vi "Main.vi"() -> ()   [LabVIEW 2017]
uses:
  type defs/action buttons.ctl
  type defs/mode buttons.ctl
  <vilib>/vision/Pattern Matching.llb/IMAQ GM Match Report.ctl
  type defs/states.ctl
  type defs/data.ctl
  <vilib>/vision/Image Controls.llb/IMAQ Image.ctl
  <vilib>/myRIO/Instrument Drivers/Onboard IO/PWM/typedefs/PWM Reference.ctl
  <vilib>/myRIO/Common/Instrument Driver Framework/Utilities/typedefs/myRIO Generic Hardware Reference.ctl
  <vilib>/myRIO/Common/Instrument Driver Framework/Utilities/typedefs/Hardware Version Enum.ctl
  <vilib>/myRIO/Common/Instrument Driver Framework/Utilities/typedefs/myRIO v1.0 Reference.ctl
  <vilib>/myRIO/Common/Instrument Driver Framework/Utilities/typedefs/Generic FPGA Reference.ctl
  <vilib>/myRIO/Common/Instrument Driver Framework/myRIO v1.0/PWM/typedefs/PWM Channels Enum.ctl
  <vilib>/myRIO/Instrument Drivers/Onboard IO/PWM/typedefs/PWM Configuration.ctl
  <vilib>/userdefined/High Color/nirio_resource_hc.ctl
  <vilib>/myRIO/Instrument Drivers/Onboard IO/DIO/typedefs/DIO Reference.ctl
  <vilib>/myRIO/Common/Instrument Driver Framework/myRIO v1.0/DIO/typedefs/DIO Channels List.ctl
  <vilib>/myRIO/Common/Instrument Driver Framework/myRIO v1.0/DIO/typedefs/DIO Channels Enum.ctl
  type defs/task.ctl
  <vilib>/myRIO/Common/Instrument Driver Framework/Utilities/vis/Is FPGA Ref Available.vi
  <vilib>/myRIO/Common/Instrument Driver Framework/myRIO v1.0/PWM/vis/myRIO v1.1 Open PWM.vi
  <vilib>/myRIO/Instrument Drivers/Onboard IO/PWM/vis/Set Duty Cycle and Frequency.vi
  <vilib>/myRIO/Common/Instrument Driver Framework/myRIO v1.0/DIO/vis/myRIO v1.1 Open DIO.vi
  <vilib>/myRIO/Instrument Drivers/Onboard IO/DIO/vis/Write.vi
  <vilib>/myRIO/Instrument Drivers/Onboard IO/DIO/vis/Read.vi
  <vilib>/myRIO/Common/Instrument Driver Framework/Utilities/vis/Validate Channels.vi
  <vilib>/myRIO/Common/Instrument Driver Framework/myRIO v1.0/PWM/vis/myRIO v1.0 Reserve PWM.vi
  <vilib>/myRIO/Common/Instrument Driver Framework/myRIO v1.0/DIO/vis/myRIO v1.0 Reserve DIO.vi
  <vilib>/myRIO/Common/Instrument Driver Framework/myRIO v1.0/UART/vis/myRIO v1.0 Close UART.vi
  <vilib>/myRIO/Common/Instrument Driver Framework/myRIO v1.0/PWM/vis/myRIO v1.0 Build MUX Configuration PWM.vi
  <vilib>/myRIO/Common/Instrument Driver Framework/myRIO v1.0/Resource Manager/vis/myRIO v1.0 Reserve Channel List.vi
  <vilib>/myRIO/Common/Instrument Driver Framework/myRIO v1.0/DIO/vis/myRIO v1.0 Build MUX Configuration DIO.vi
  <vilib>/myRIO/Common/Instrument Driver Framework/myRIO v1.0/Resource Manager/vis/myRIO v1.0 Create Configuration List.vi
  <vilib>/myRIO/Common/Instrument Driver Framework/myRIO v1.0/Resource Manager/vis/myRIO v1.0 Reserve Channel.vi
  <vilib>/myRIO/Common/Instrument Driver Framework/myRIO v1.0/Resource Manager/vis/myRIO v1.0 Unreserve Channel.vi
  <vilib>/myRIO/Common/Instrument Driver Framework/myRIO v1.0/Resource Manager/vis/myRIO v1.0 Build Mutex Name.vi
  <vilib>/Utility/VariantDataType/GetNumericInfo.vi
  <vilib>/Utility/error.llb/Error Cluster From Error Code.vi
  <vilib>/myRIO/Common/Instrument Driver Framework/myRIO v1.0/myRIO v1.1 Open.vi
  <vilib>/myRIO/Common/Instrument Driver Framework/Utilities/vis/IO Manager.vi
  <vilib>/myRIO/Common/Instrument Driver Framework/Utilities/vis/Configuration Manager.vi
  <vilib>/myRIO/Common/Instrument Driver Framework/myRIO v1.0/Resource Manager/vis/myRIO v1.0 Configure IO.vi
  <vilib>/myRIO/Common/Instrument Driver Framework/myRIO v1.0/myRIO v1.0 Close.vi
  <vilib>/myRIO/Common/Instrument Driver Framework/myRIO v1.0/PWM/vis/myRIO v1.0 Write PWM.vi
  <vilib>/myRIO/Common/Instrument Driver Framework/myRIO v1.0/DIO/vis/myRIO v1.0 Write DIO.vi
  <vilib>/myRIO/Common/Instrument Driver Framework/myRIO v1.0/DIO/vis/myRIO v1.0 Read DIO.vi
  <vilib>/myRIO/Common/Instrument Driver Framework/Utilities/vis/FPGA Ref Manager.vi
  <vilib>/myRIO/Common/Instrument Driver Framework/myRIO v1.0/myRIO v1.0 Reset FPGA.vi
  <vilib>/myRIO/Common/Instrument Driver Framework/myRIO v1.0/IRQ/vis/myRIO v1.0 IRQ Info FGV.vi
  <vilib>/myRIO/Common/Instrument Driver Framework/myRIO v1.0/IRQ/vis/myRIO v1.0 Timer IRQ Info FGV.vi
  <vilib>/myRIO/Common/Instrument Driver Framework/myRIO v1.0/IRQ/vis/myRIO v1.0 ISR Agent.vi
  <vilib>/myRIO/Express VI/Onboard IO/PWM/PWM Express VI.xnode
  <vilib>/myRIO/Instrument Drivers/Onboard IO/PWM/vis/myRIO PWM Open.xnode
  <vilib>/myRIO/Express VI/Onboard IO/DO/DO Express VI.xnode
  <vilib>/myRIO/Instrument Drivers/Onboard IO/DIO/vis/myRIO DIO Open.xnode
  <vilib>/myRIO/Express VI/Onboard Devices/LED/LED Express VI.xnode
  <vilib>/myRIO/Express VI/Onboard Devices/Button/Button Express VI.xnode
  <vilib>/vision/NI_Vision_Development_Module.lvlib
  <vilib>/myRIO/Instrument Drivers/Onboard IO/DIO/DIO.lvlib
  <vilib>/myRIO/Instrument Drivers/Onboard IO/PWM/PWM.lvlib
  <vilib>/myRIO/Instrument Drivers/Utilities/Utilities.lvlib
panel:
  in  "Ball index":i32
  in  "sensivity":dbl=35000.0 format="%#_13g"
  in  "ROI Descriptor COLOR Mask":T1={"Global Rectangle"=[0, 0, 0, 0], "Contours"=[{"ID"=enum."External", "Type"=0, "Coordinates"=[0, 0, 0, 0]}]}
  out "Radius (circle)":dbl
  out "y0 (circle)":i32
  out "x0 (circle)":i32
  out "x1 (circle)":i32
  out "y1 (circle)":i32
  in  "divider (circle)":sgl=1.0
  out "CircleRadius":dbl
  in  "Look at ball":bool
  in  "x = y?":bool
  in  "y":sgl=1.0
  out "Scale":sgl
  out "error out":errorcluster
  in  "Tab Control":enum32{"Motors", "Shape/Color", "Pattern"}(tab)
  in  "Left+":bool
  in  "Left-":bool
  in  "Right+":bool
  in  "Right-":bool
  in  "M+":bool
  in  "M-":bool
  in  "G+":bool
  in  "G-":bool
  in  "M_PWM":dbl=0.5
  in  "L_PWM":dbl=0.5
  in  "R_PWM":dbl=0.5
  in  "M+ (onGrab)":bool
  out "Circles Calibrated (Shape Detection 1)":T2(array[cluster]) {"Position"."Y" format="%.2f"; "Position"."X" format="%.2f"}
  out "Number of Matches (Shape Detection 1)":i32
  out "Color":i32
  in  "Circle Descriptor (Shape Detection 1)":cluster{"Min Radius":dbl, "Max Radius":dbl}={"Min Radius"=16.0, "Max Radius"=500.0}
  in  "Align X - t, Y - f":bool
  in  "grab time (ms)":u32
  out "Class (Particle Classification 1)":string
  out "y0":i32
  out "x0":i32
  out "x1":i32
  out "y1":i32
  out "Number of Matches (Geometric Matching 1)":i32
  out "Calibrated Matches (Geometric Matching 1)":T3[](array[typedef]) {"Correlation Score" format="%.2f"; "Target Template Curve Score" format="%.2f"; "Template Target Curve Score" format="%.2f"; "Bounding Box"."y" format="%.2f"; "Bounding Box"."x" format="%.2f"; "Position"."y" format="%.2f"; "Position"."x" format="%.2f"; "Score" format="%.2f"; "Scale" format="%.2f"; "Angle" format="%.2f"; "Occlusion %" format="%.2f"}
  out "curY":sgl
  out "curX":sgl
  out "Y is in range":bool
  out "X is in range":bool
  in  "defY":dbl=170.0
  in  "Range":dbl=40.0
  in  "defX":dbl=150.0
  in  "mode buttons":T4
  out "image display":T5(plugin-control)
  in  "action buttons":T6
  in  "Stop":bool
  # "Machine\nVision\nApp"
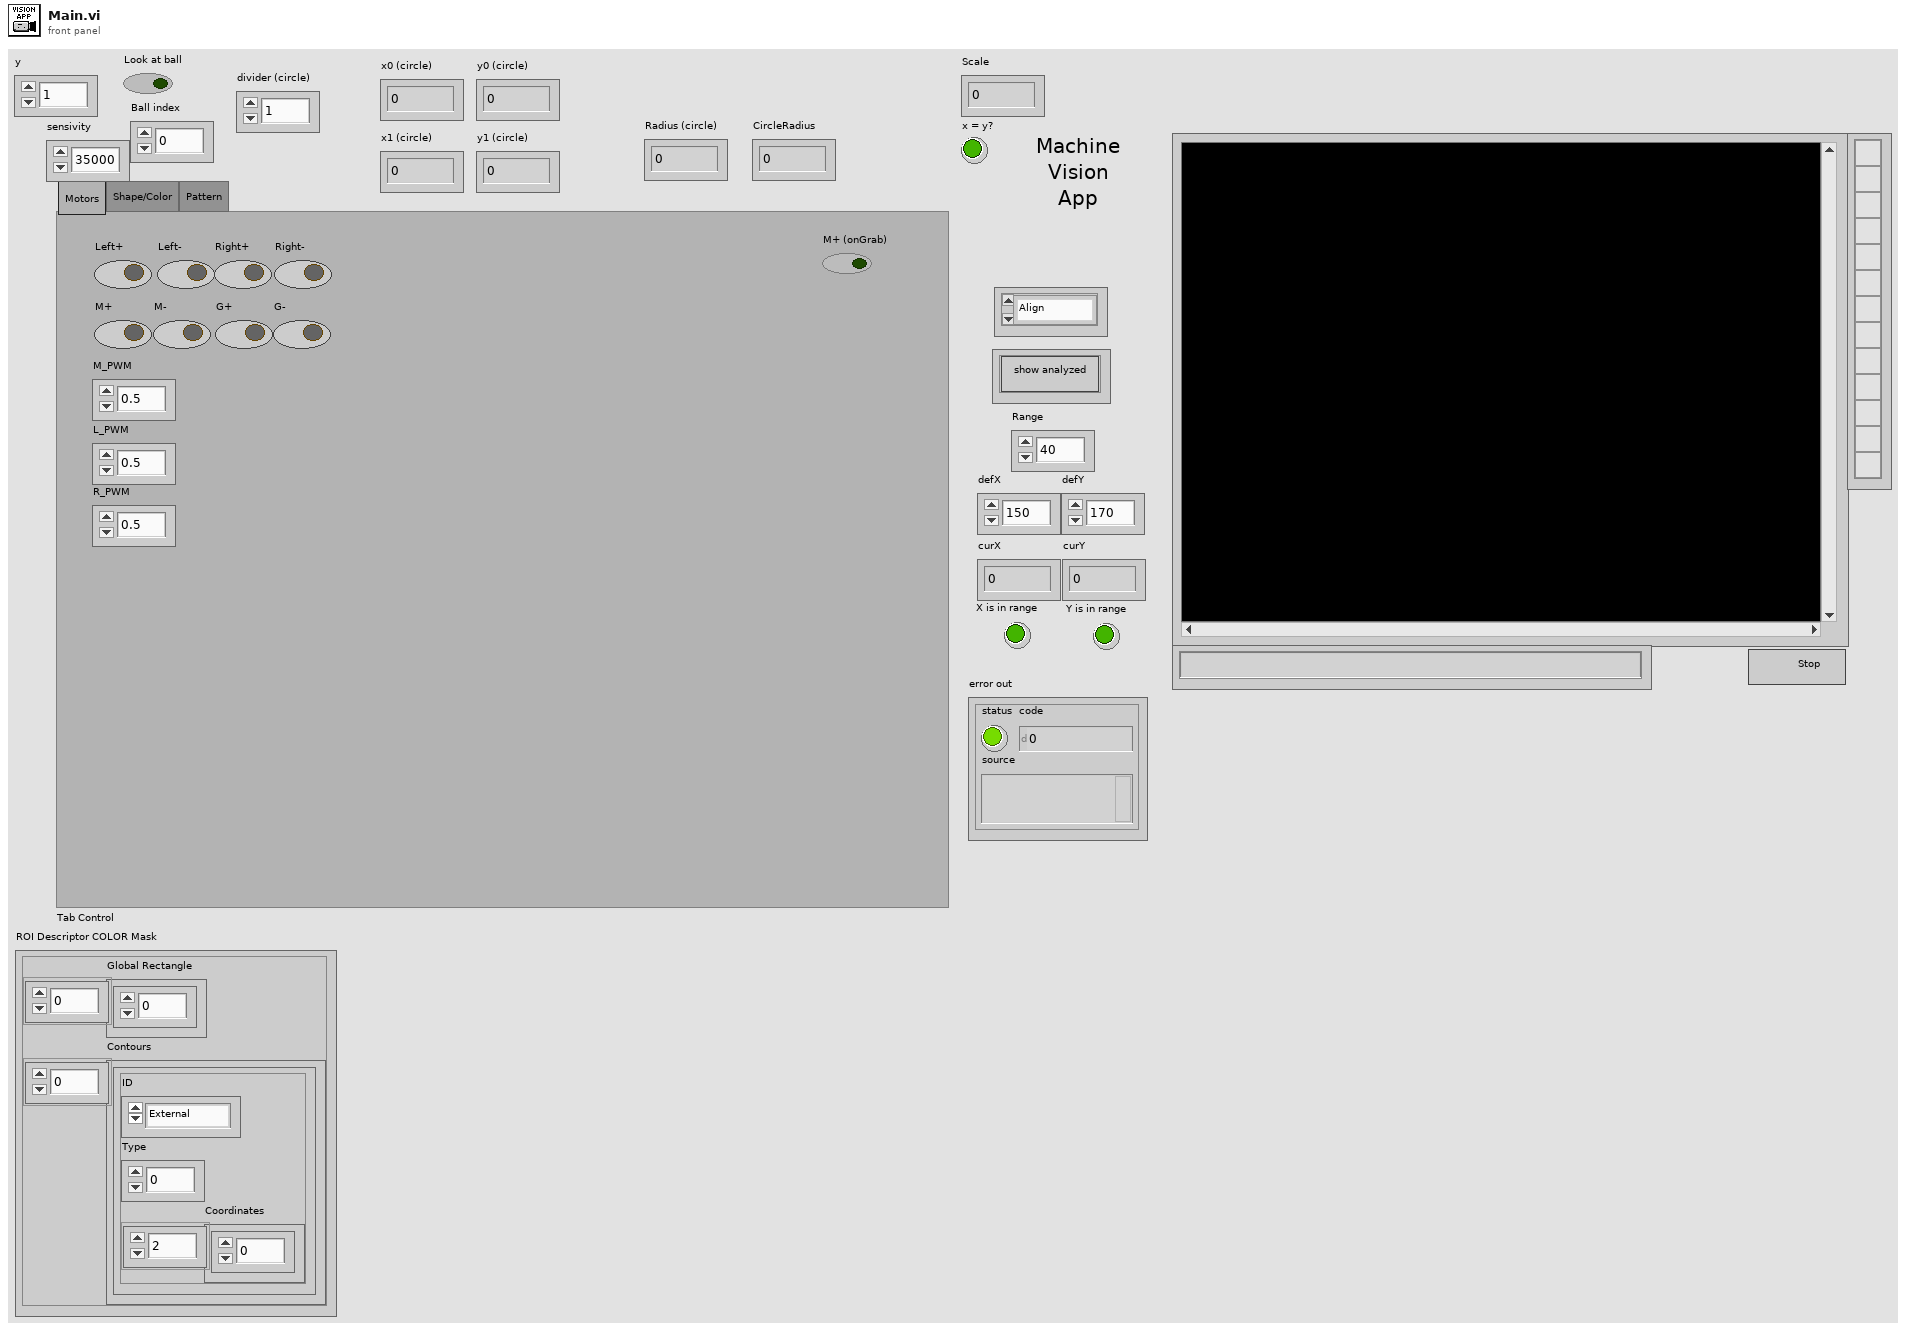
[diagram p1: front panel]
types:
  T1 = cluster{"Global Rectangle":i32[], "Contours":cluster{"ID":enum32{"External", "Internal"}, "Type":u32, "Coordinates":i32[]}[]}
  T2 = cluster{"Position":cluster{"X":sgl, "Y":sgl}, "Radius":dbl, "Score":dbl}[]
  T3 = typedef "IMAQ GM Match Report.ctl" = cluster{"Position":cluster{"x":sgl, "y":sgl}, "Angle":sgl, "Scale":sgl, "Score":sgl, "Bounding Box":cluster{"x":sgl, "y":sgl}[], "Contrast Reversed":bool, "Occlusion %":sgl, "Template Target Curve Score":sgl, "Target Template Curve Score":sgl, "Correlation Score":sgl}
  T4 = typedef "mode buttons.ctl" = cluster{"show analyzed":bool}
  T5 = typedef "IMAQ Image.ctl" = refnum<image>
  T6 = typedef "action buttons.ctl" = cluster{"Shape - t, Color - f":enum16{"Align", "Pattern", "Ball", "Other", "Clear", "Joystick control"}}
  T7 = typedef "states.ctl" = enum16{"(qsm) schedule", "(qsm) initialize", "(qsm) release", "(qsm) clean up", "(qsm) shutdown", "(myRIO) initialize", "(myRIO) clean up", "(myRIO) update ports", "(image) get", "(image) analyze", "(image) show", "(ball) Shape detection", "(ball) Calc ball indx", "(ball) Calculate ROI", "X align", "Wait", "Grab", "(pattern) Find Square", "(pattern) Calculate ROI", "(pattern) Analyze pattern", "(joystick) Joystick control", "Wait for button"}
  T8 = typedef "DIO.lvlib/DIO Reference.ctl" = cluster{"myRIO Reference":T9, "DIO Channels List":T13}
  T9 = typedef "myRIO Generic Hardware Reference.ctl" = cluster{"myRIO Model":T10, "myRIO Hardware Reference":T11}
  T10 = typedef "Hardware Version Enum.ctl" = enum16{"Unknown", "myRIO-1900", "myRIO-1950", "roboRIO", "NI ELVIS RIO CM"}
  T11 = typedef "myRIO v1.0 Reference.ctl" = cluster{"Generic FPGA Reference":T12, "Allow multiple opens":bool}
  T12 = typedef "Generic FPGA Reference.ctl" = refnum<k20>
  T13 = typedef "DIO Channels List.ctl" = T14[]
  T14 = typedef "DIO Channels Enum.ctl" = enum16{"Not Connected", "C/DIO0", "C/DIO1", "C/DIO2", "C/DIO3", "C/DIO4", "C/DIO5", "C/DIO6", "C/DIO7", "A/DIO0", "A/DIO1", "A/DIO2", "A/DIO3", "A/DIO4", "A/DIO5", "A/DIO6", "A/DIO7", "A/DIO8", "A/DIO9", "A/DIO10", "A/DIO11", "A/DIO12", "A/DIO13", "A/DIO14", "A/DIO15", "B/DIO0", "B/DIO1", "B/DIO2", "B/DIO3", "B/DIO4", "B/DIO5", "B/DIO6", "B/DIO7", "B/DIO8", "B/DIO9", "B/DIO10", "B/DIO11", "B/DIO12", "B/DIO13", "B/DIO14", "B/DIO15", "LED0", "LED1", "LED2", "LED3", "Button0", "DIO/DIO0", "DIO/DIO1", "DIO/DIO2", "DIO/DIO3", "DIO/DIO4", "DIO/DIO5", "DIO/DIO6", "DIO/DIO7", "DIO/DIO8", "DIO/DIO9", "SPI/CS0", "SPI/CS1", "SPI/CS2", "SPI/CS3", "LED RADIO (Green)", "LED RADIO (Red)", "LED COMM (Green)", "LED COMM (Red)", "LED MODE (Green)", "LED MODE (Red)"}
  T15 = typedef "nirio_resource_hc.ctl" = tag
  T16 = typedef "PWM.lvlib/PWM Reference.ctl" = cluster{"myRIO Reference":T9, "PWM Channels Enum":T17, "PWM Configuration":T18}
  T17 = typedef "PWM Channels Enum.ctl" = enum16{"Not Connected", "C/PWM0", "C/PWM1", "A/PWM0", "A/PWM1", "A/PWM2", "B/PWM0", "B/PWM1", "B/PWM2", "PWM/PWM0", "PWM/PWM1", "PWM/PWM2", "PWM/PWM3", "PWM/PWM4", "PWM/PWM5", "PWM/PWM6", "PWM/PWM7", "PWM/PWM8", "PWM/PWM9"}
  T18 = typedef "PWM.lvlib/PWM Configuration.ctl" = cluster{"Frequency":dbl, "Duty Cycle":dbl}
  T19 = typedef "data.ctl" = cluster{"Shape - t, Color - f":bool, "qsm":cluster{"Webcam image ref":T5, "Analyzed image ref":T5, "Stop webcam":bool}, " image ref":T5, "number img":i32, "ROI Descriptor (Image Mask 1)":cluster{"Global Rectangle":i32[], "Contours":cluster{"ID":enum32{"External", "Internal"}, "Type":u32, "Coordinates":i32[]}[]}, "Pattern class":i32, "Color class":i32[], "ROI Descriptor COLOR Mask":cluster{"Global Rectangle":i32[], "Contours":cluster{"ID":enum32{"External", "Internal"}, "Type":u32, "Coordinates":i32[]}[]}}
  T20 = enum16{"Align", "Pattern", "Ball", "Other", "Clear", "Joystick control"}
  T21 = typedef "task.ctl" = T7[]
  T22 = typedef "Image Type" = u32
  T23 = cluster{"Position":cluster{"X":sgl, "Y":sgl}, "Radius":dbl, "Score":dbl}
  T24 = cluster{"ID":enum32{"External", "Internal"}, "Type":u32, "Coordinates":i32[]}[]
  T25 = cluster{"ID":enum32{"External", "Internal"}, "Type":u32, "Coordinates":i32[]}
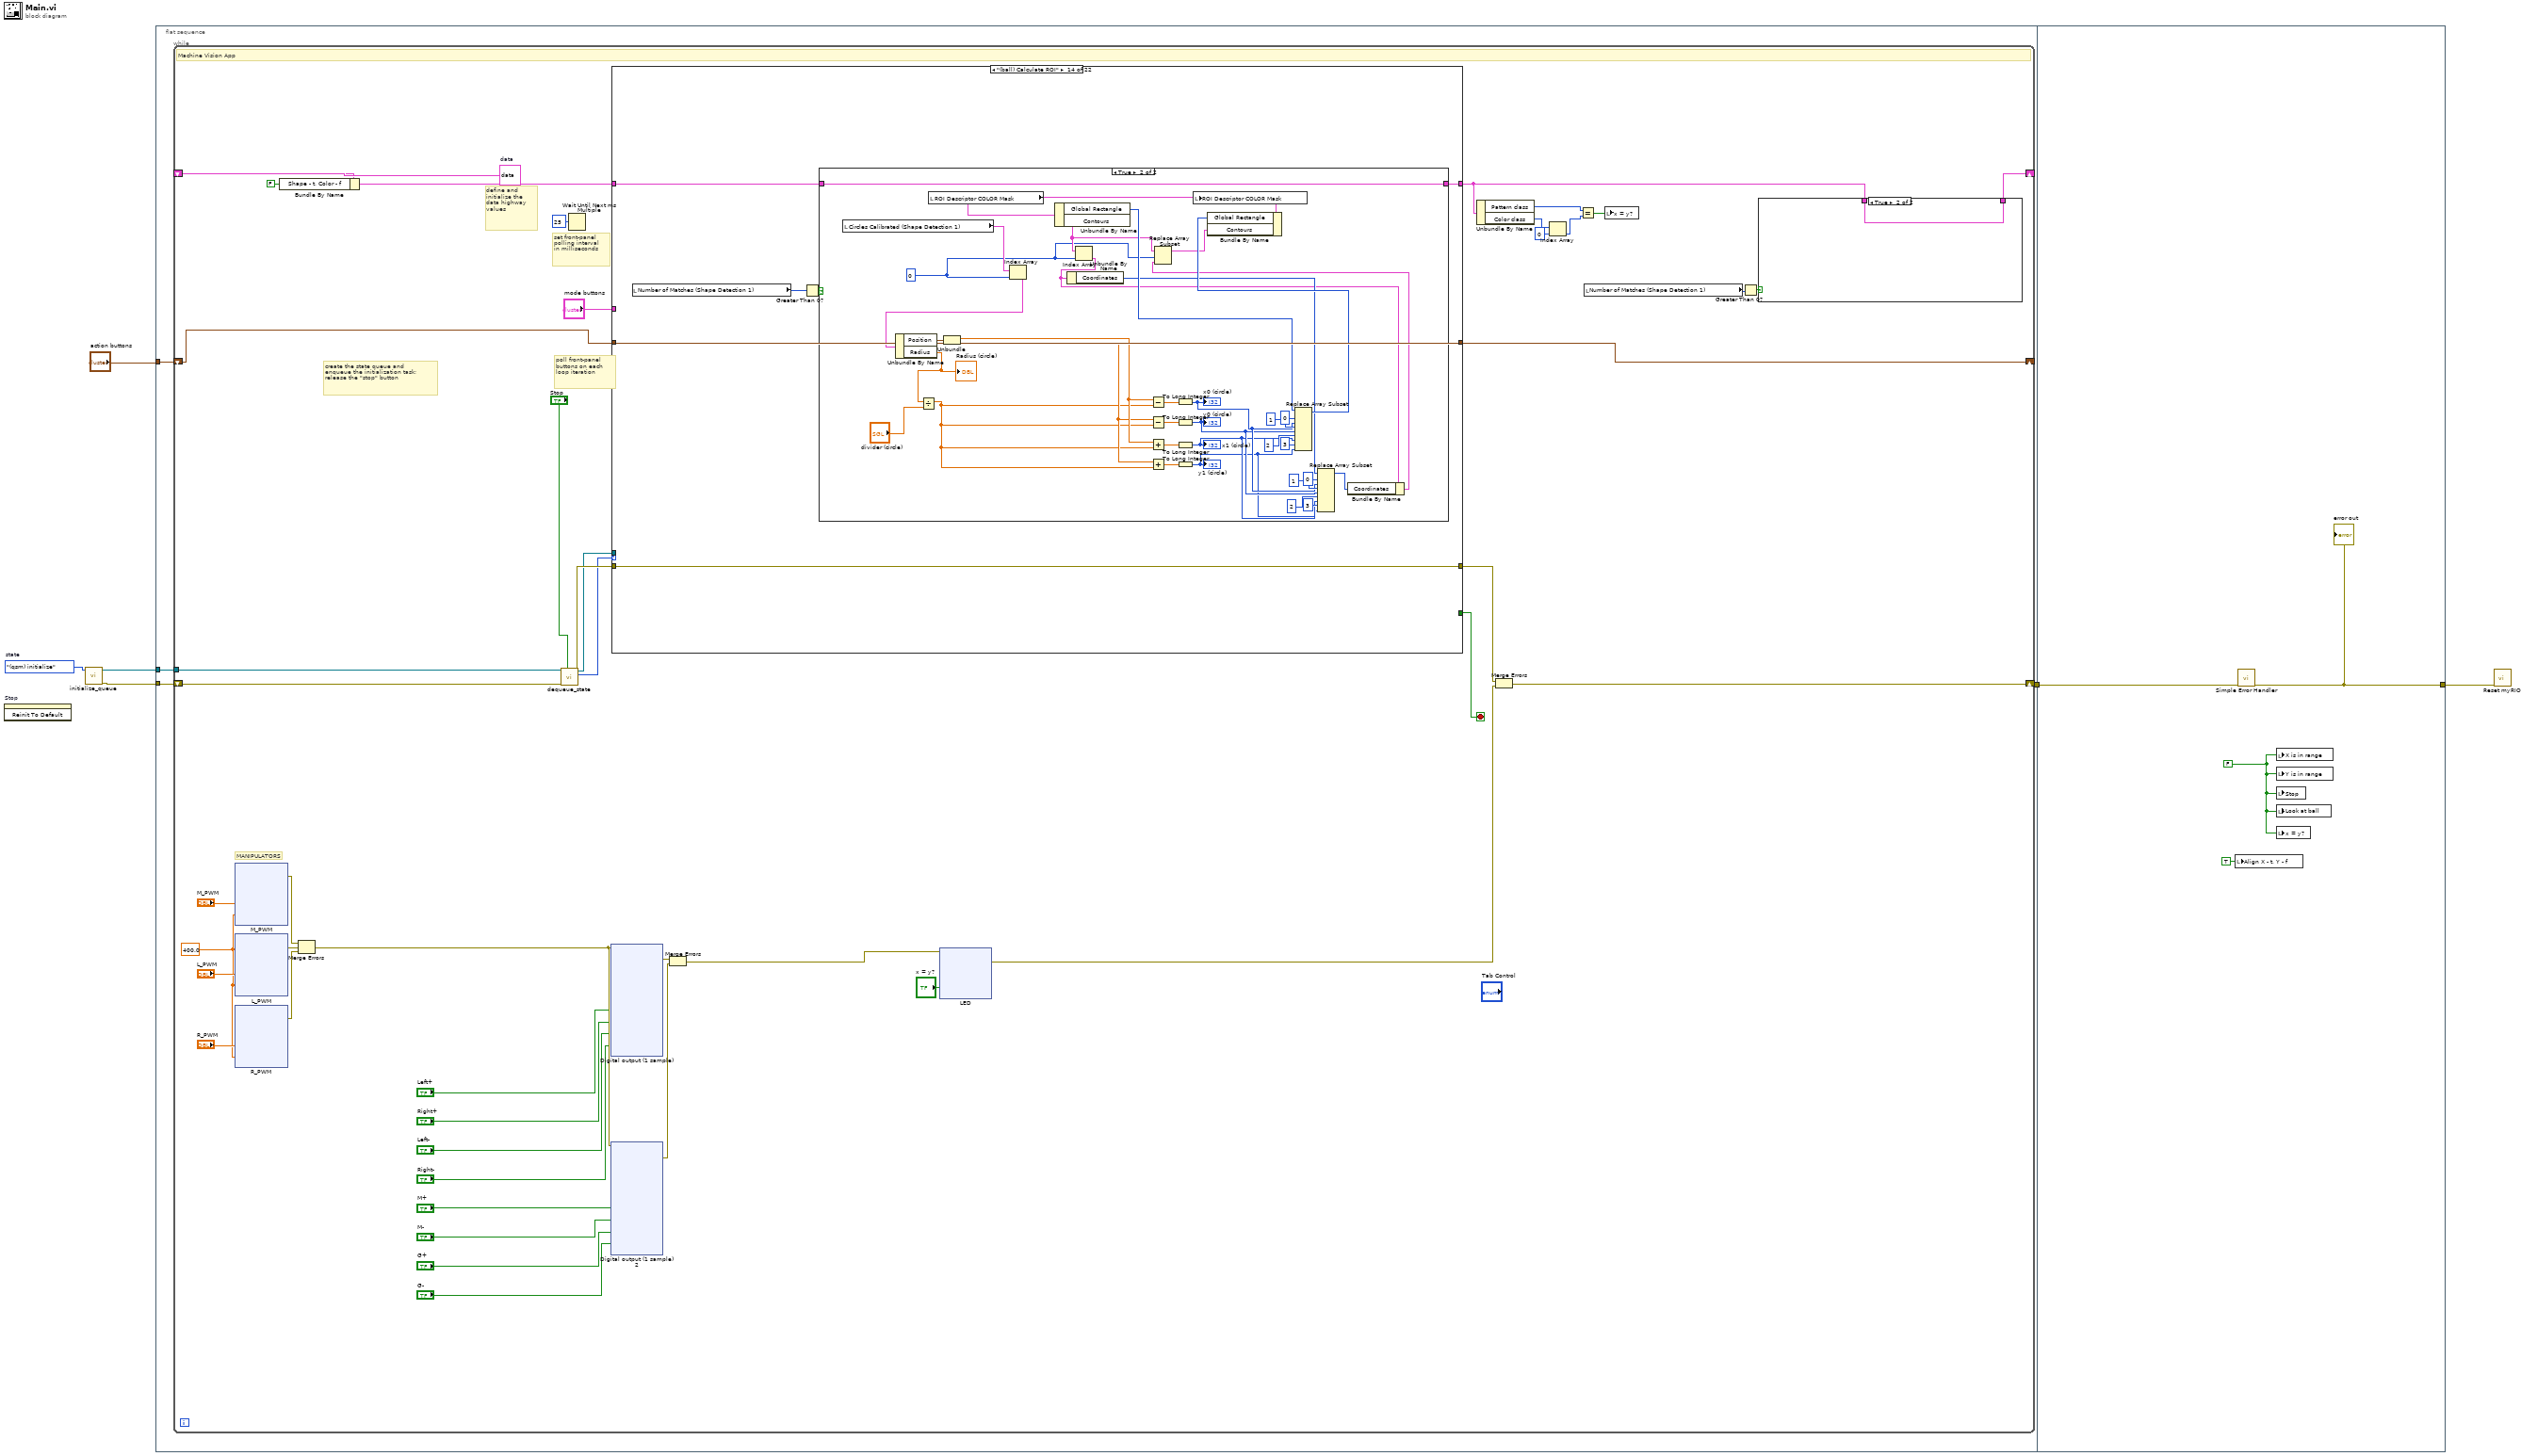
[diagram p0: block diagram]
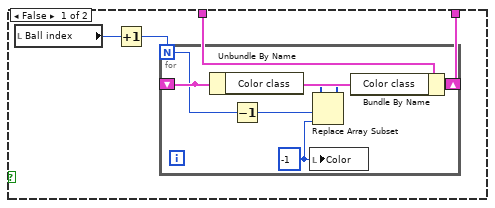
[diagram p2: hidden frame]
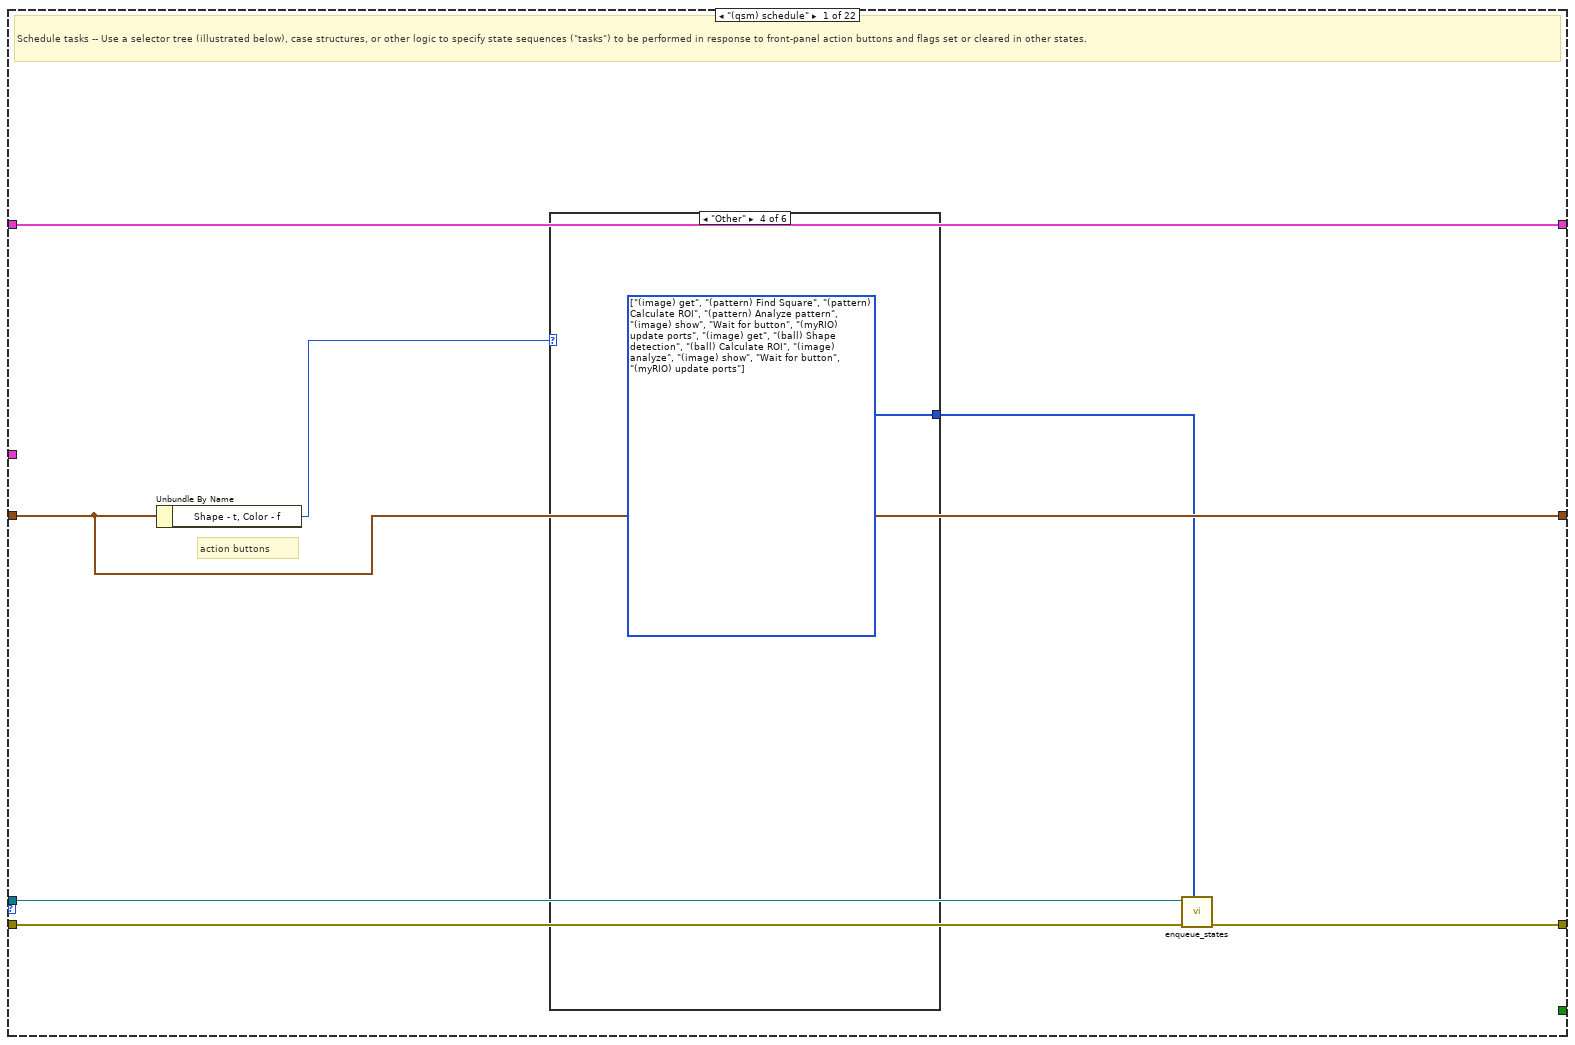
[diagram p3: hidden frame]
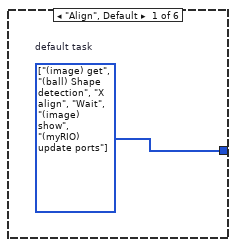
[diagram p4: hidden frame]
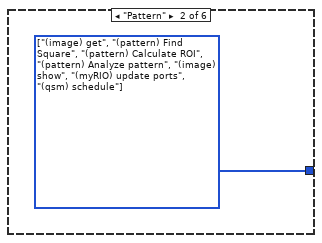
[diagram p5: hidden frame]
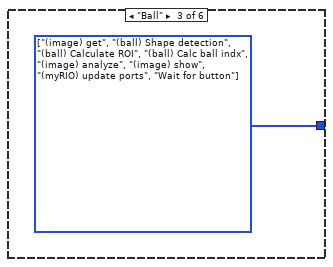
[diagram p6: hidden frame]
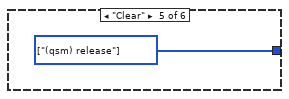
[diagram p7: hidden frame]
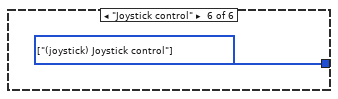
[diagram p8: hidden frame]
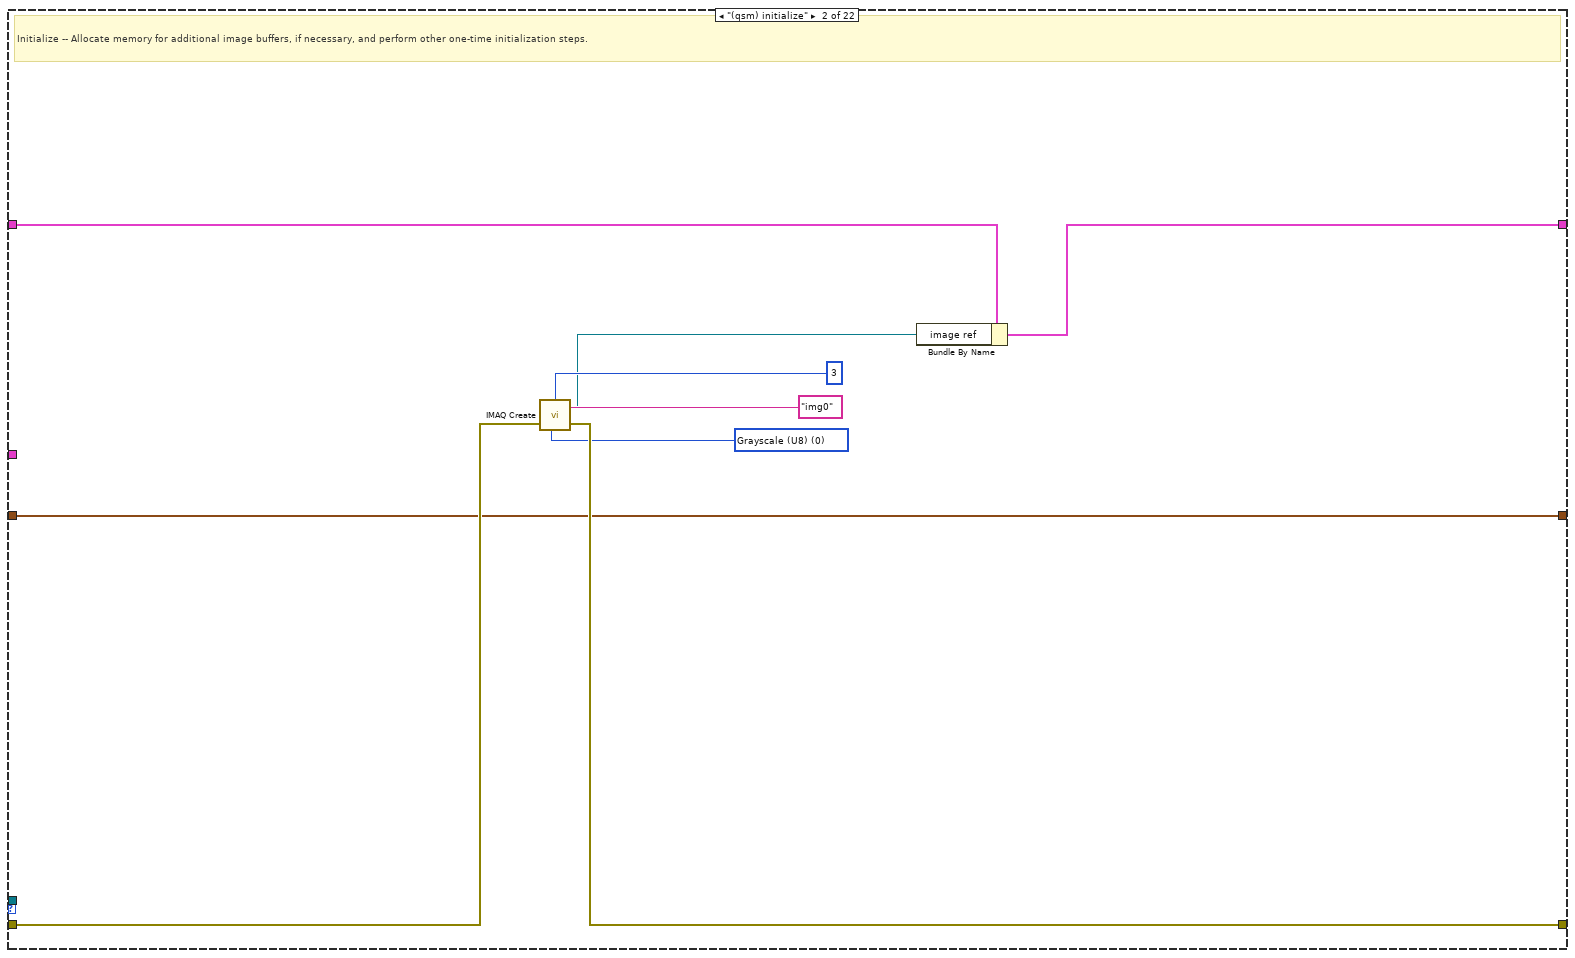
[diagram p9: hidden frame]
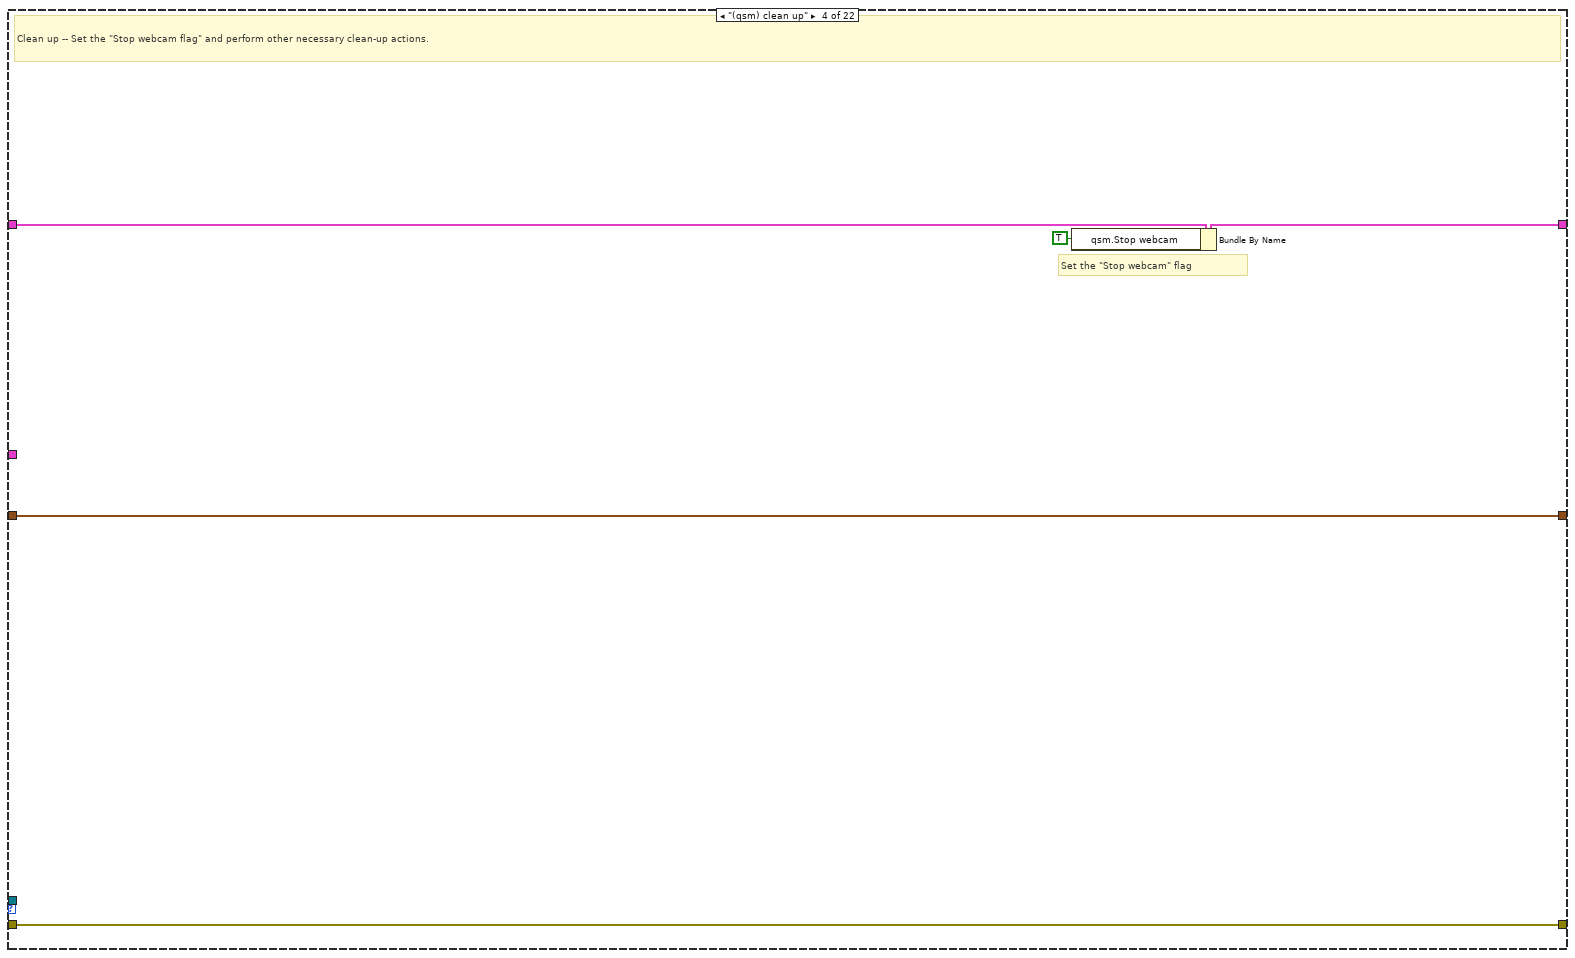
[diagram p11: hidden frame]
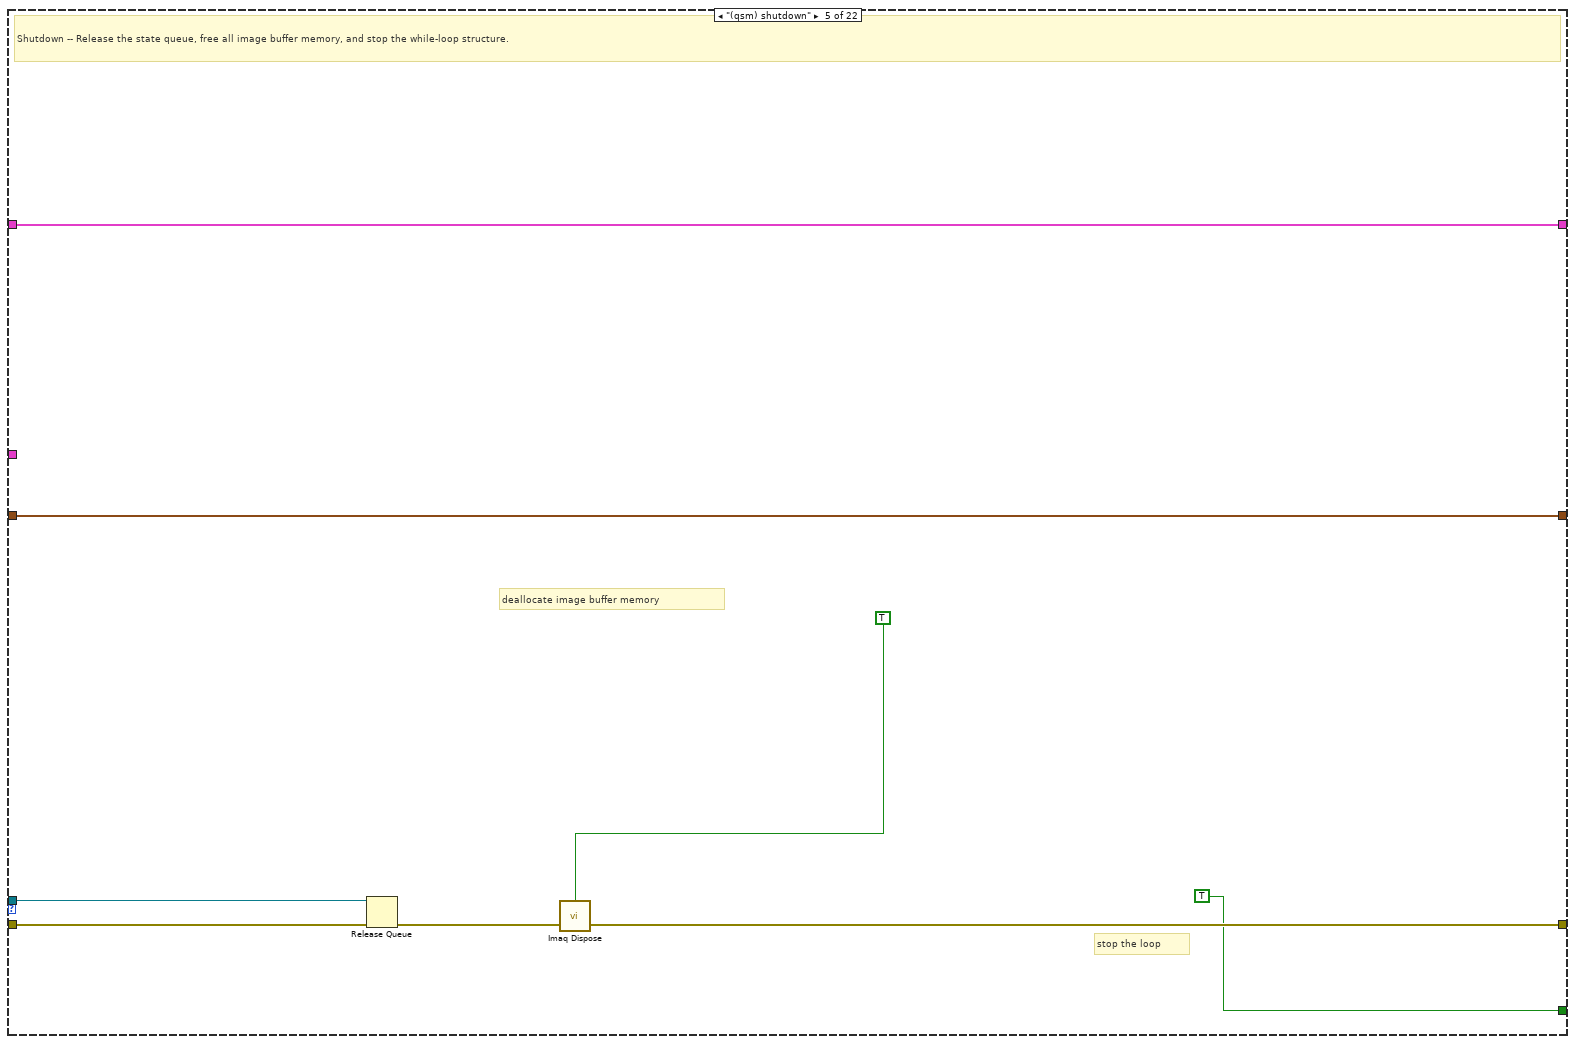
[diagram p12: hidden frame]
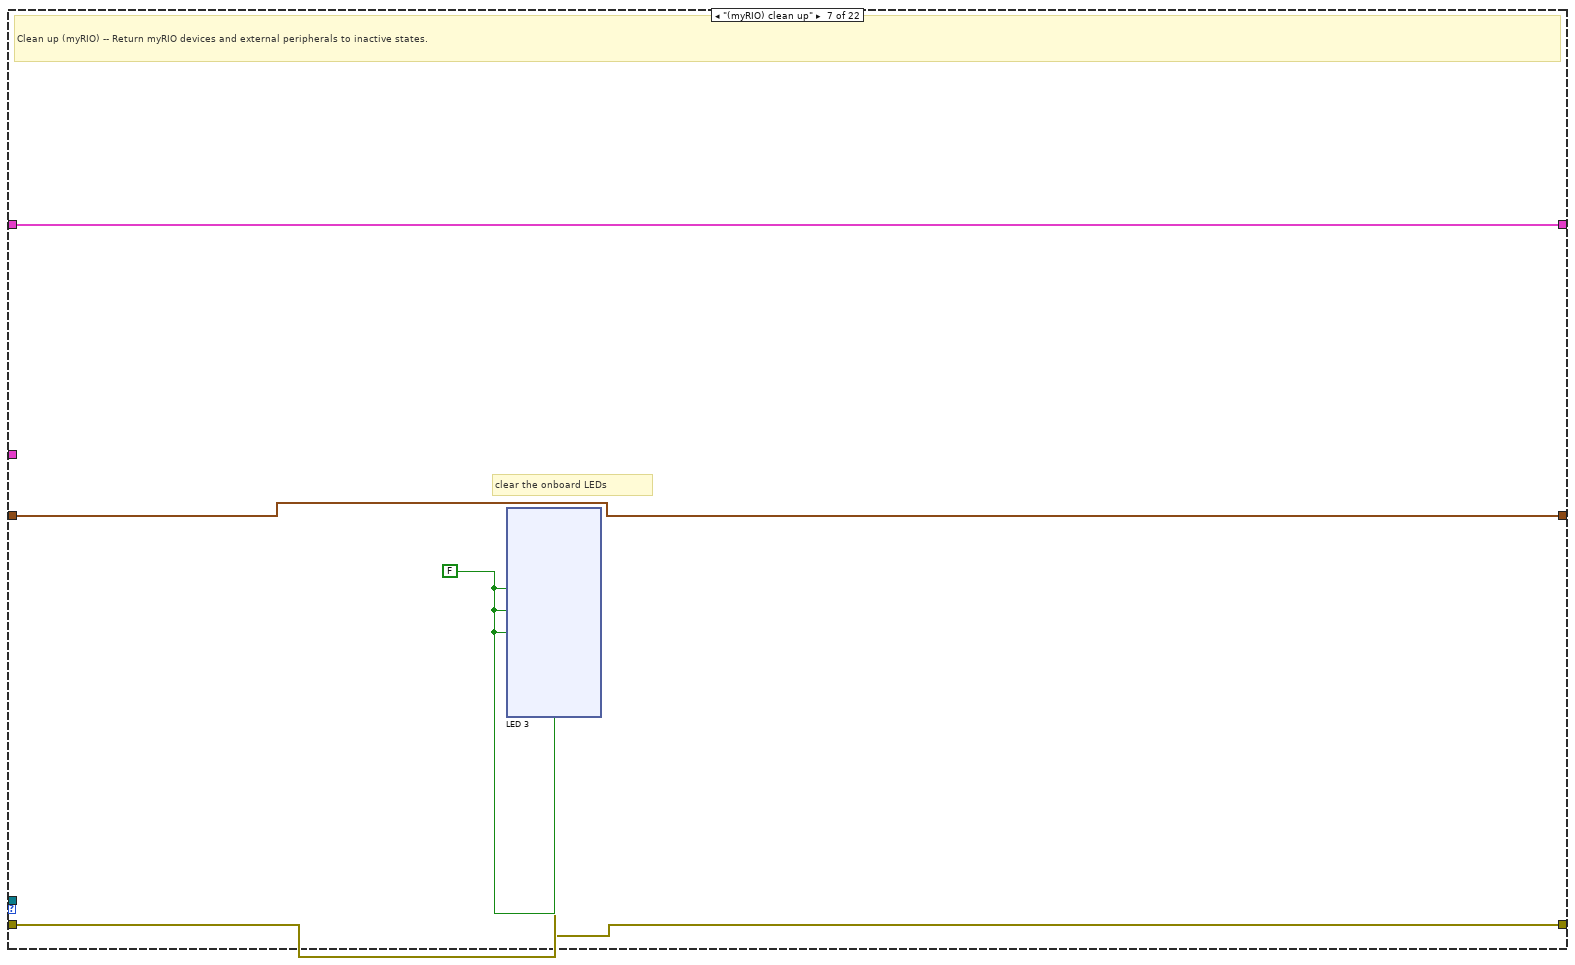
[diagram p14: hidden frame]
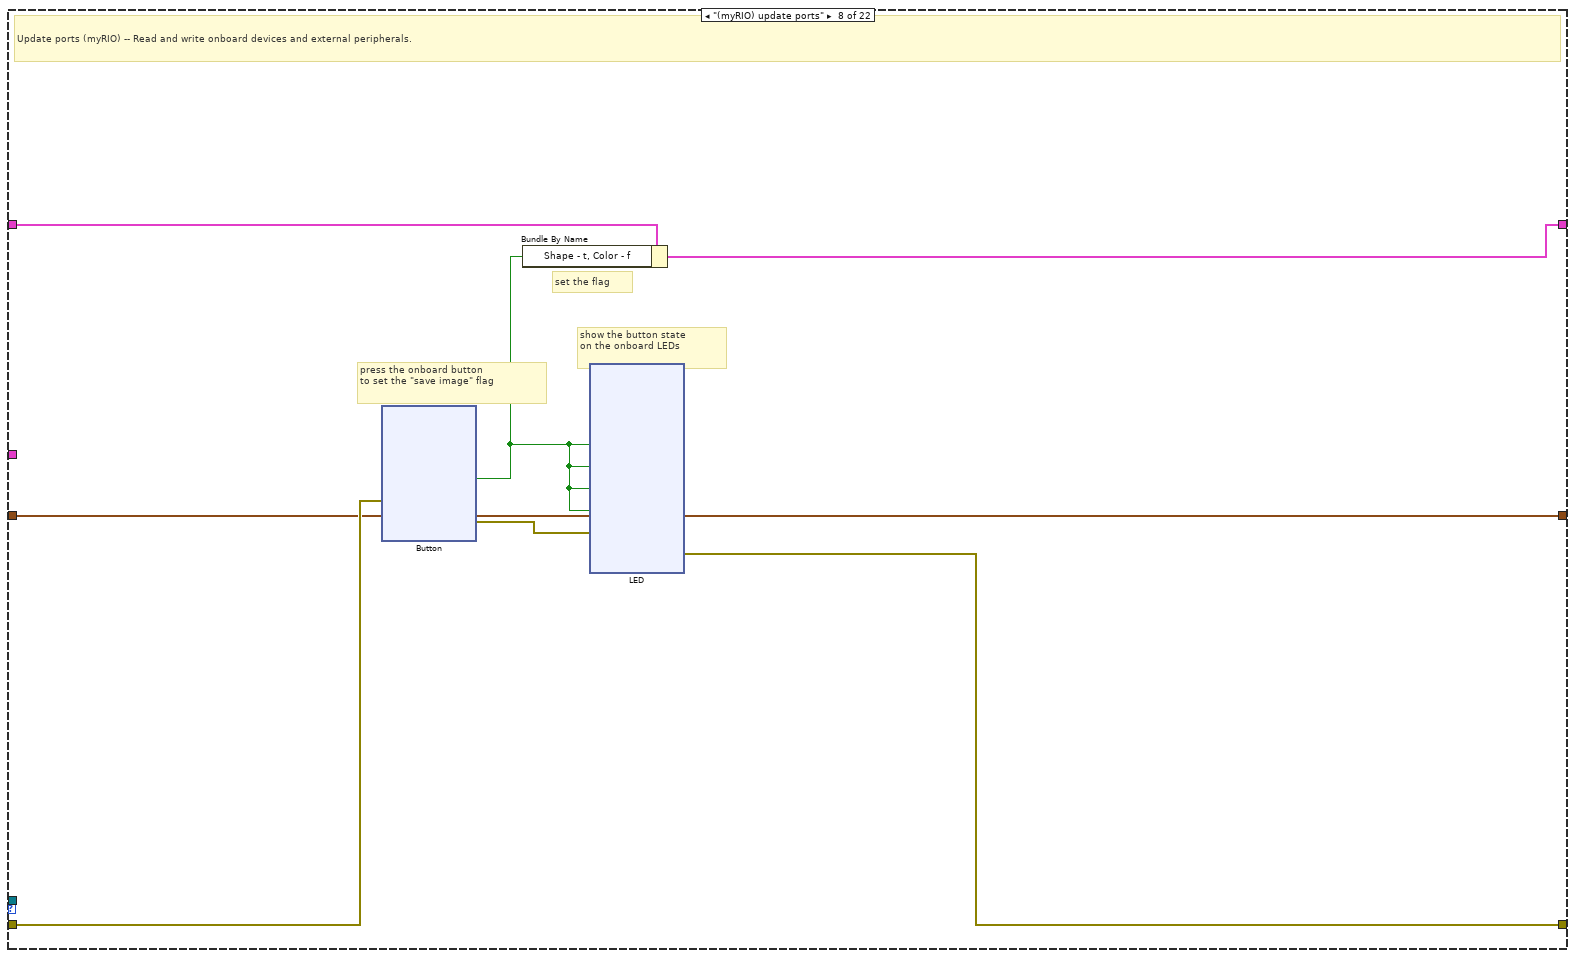
[diagram p15: hidden frame]
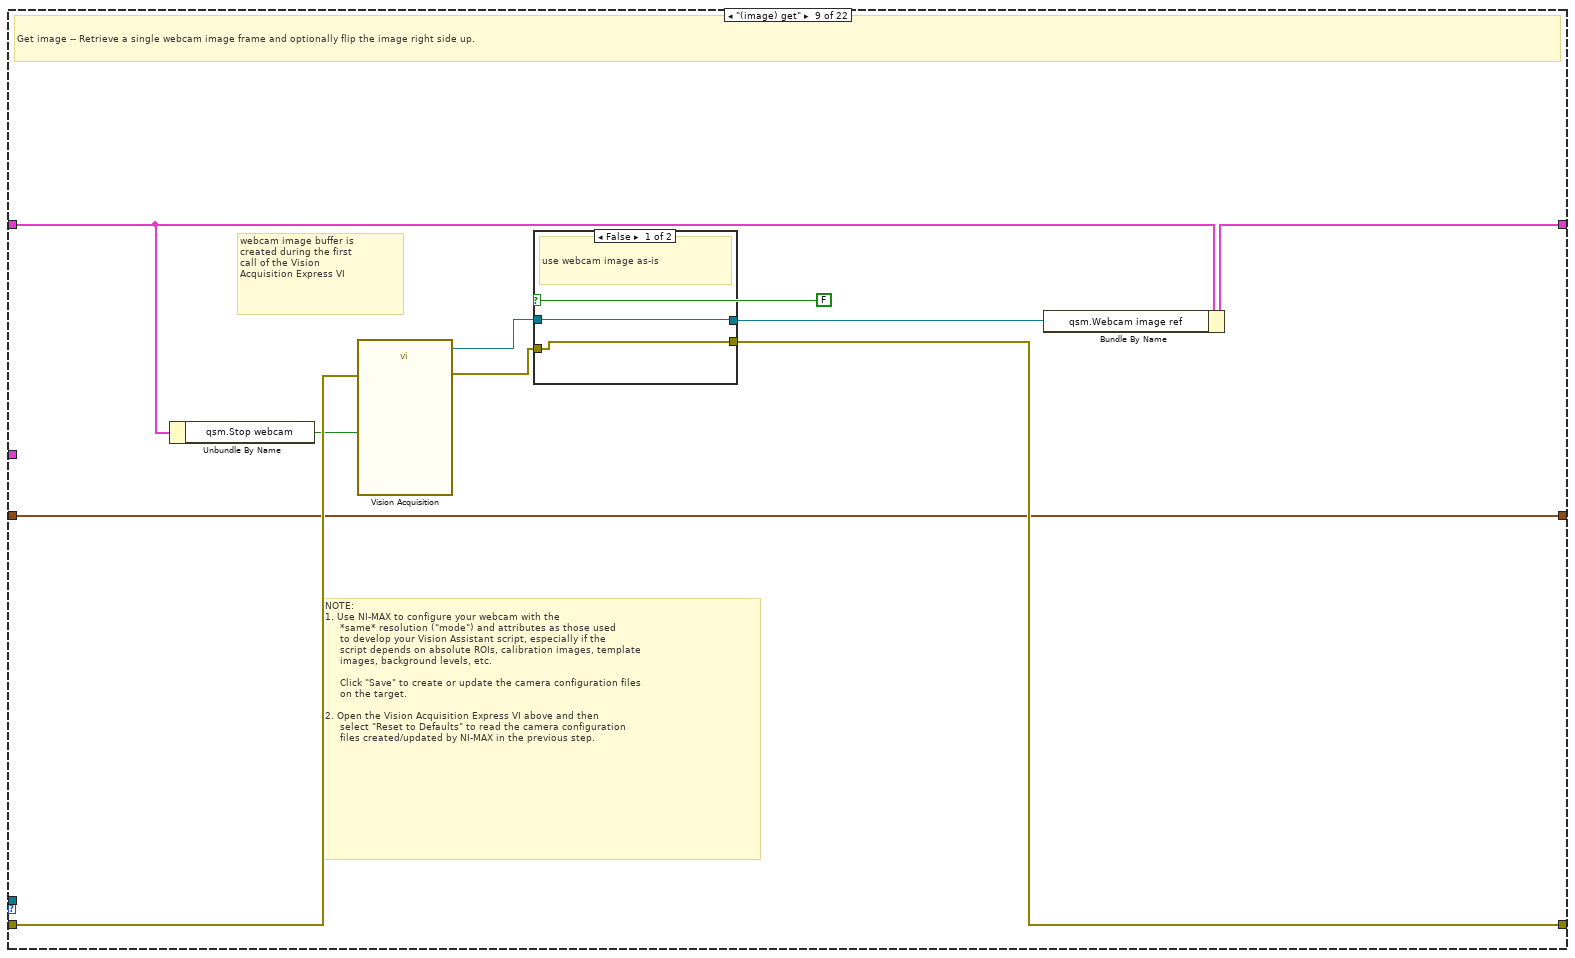
[diagram p16: hidden frame]
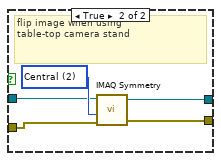
[diagram p17: hidden frame]
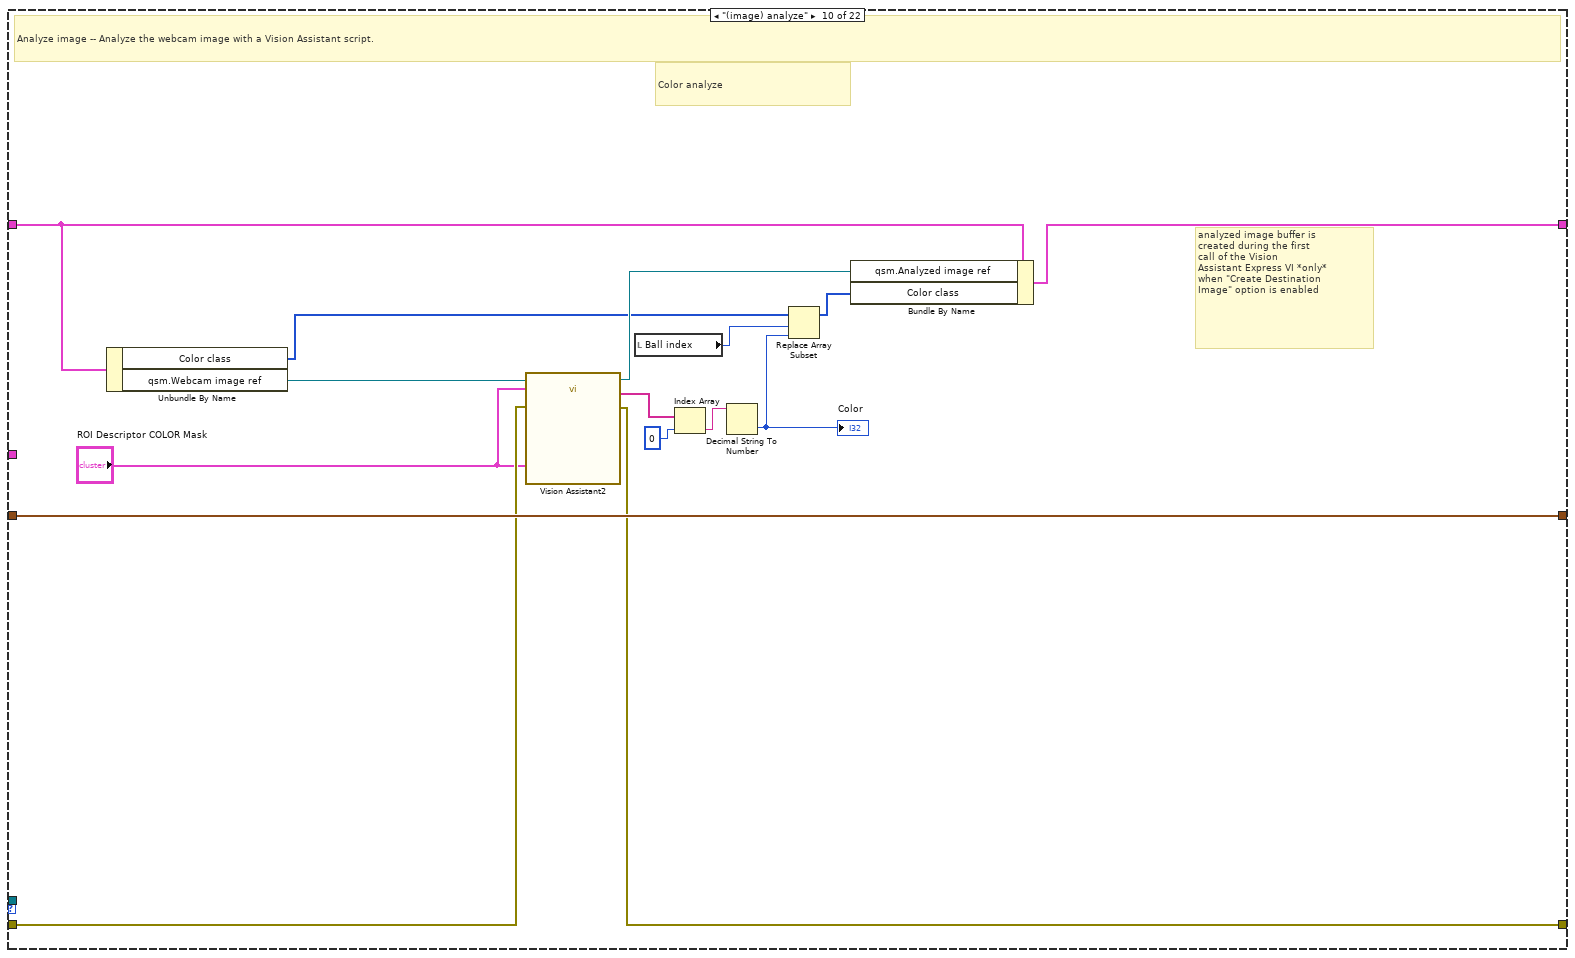
[diagram p18: hidden frame]
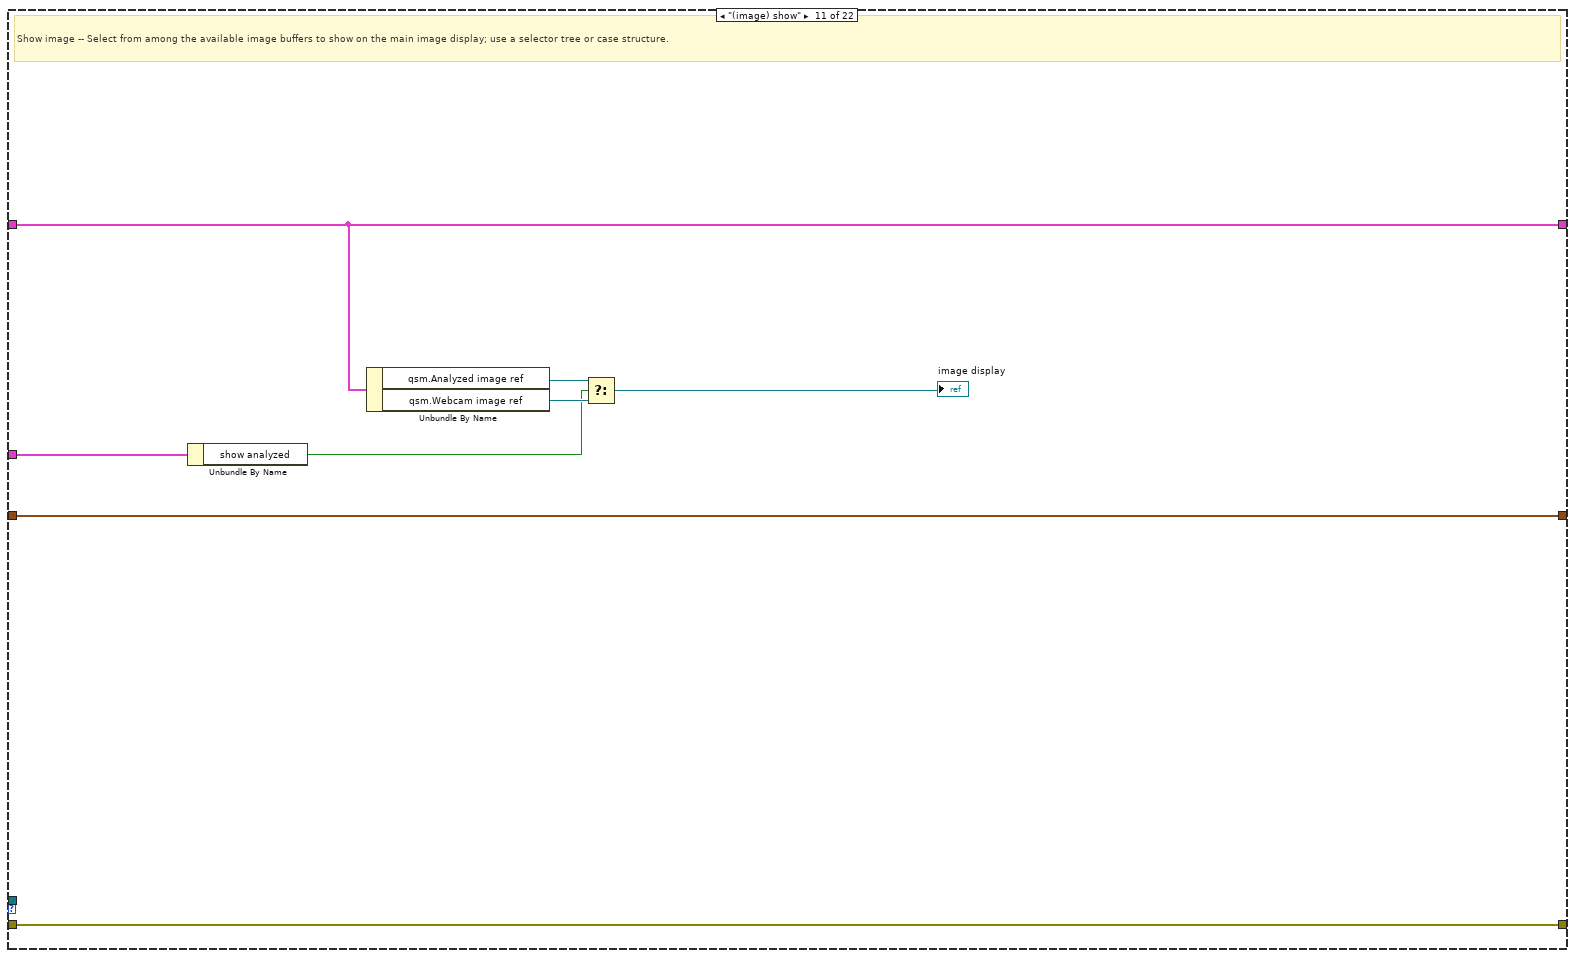
[diagram p19: hidden frame]
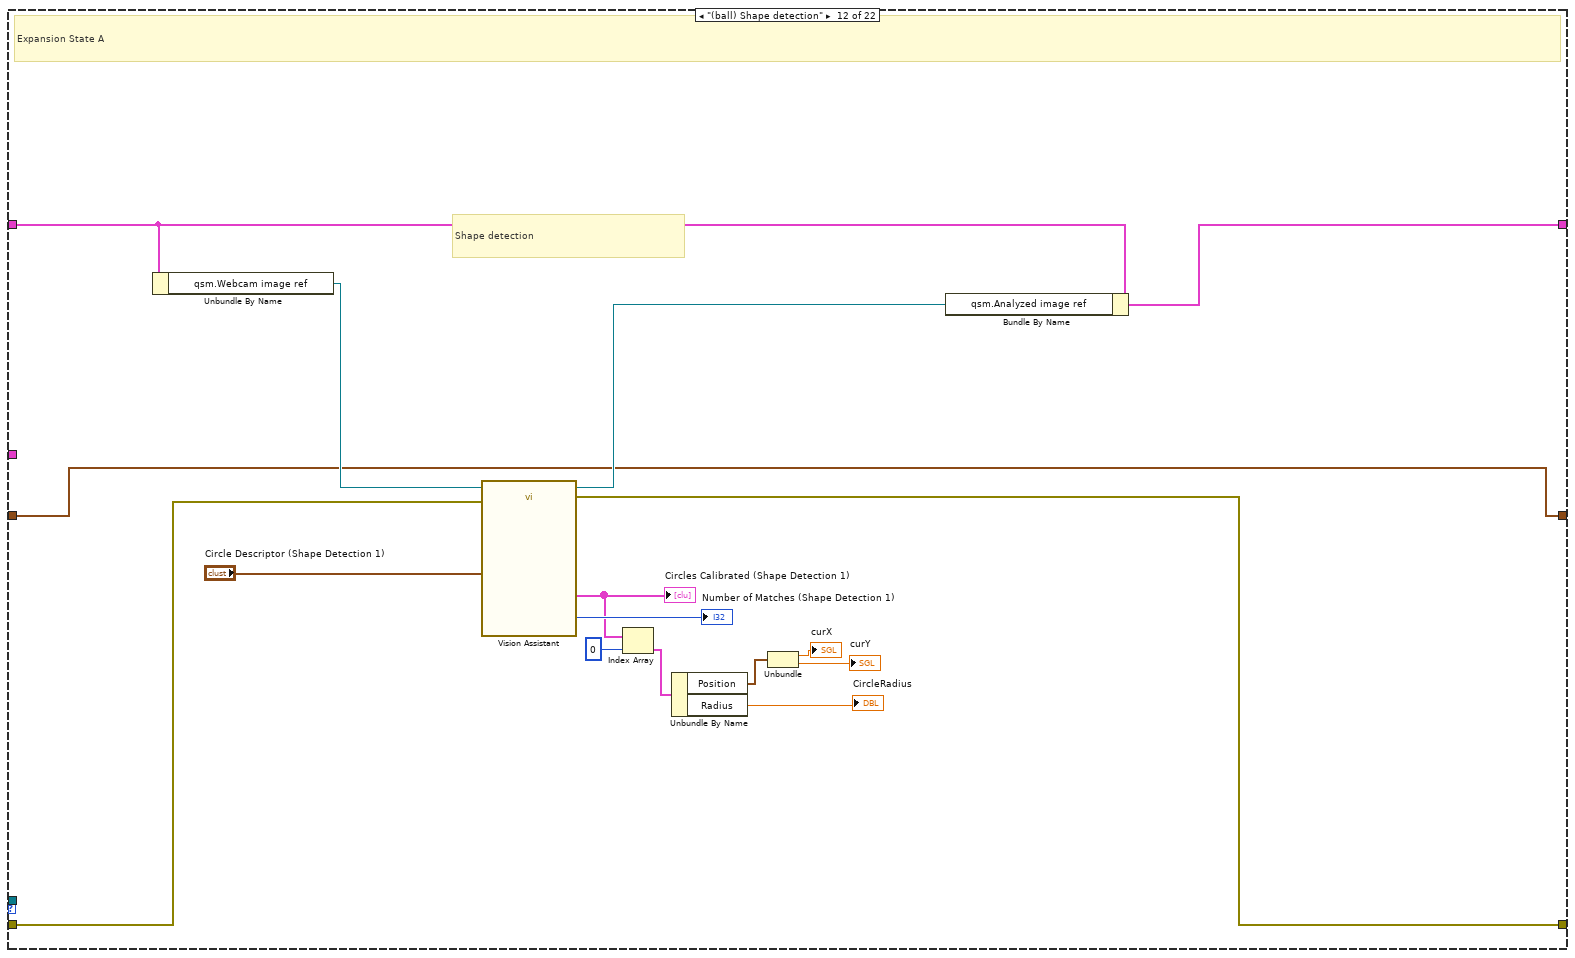
[diagram p20: hidden frame]
diagram:
  w1 = states."(qsm) initialize"  # state
  n1 = invoke on="Stop" class="Bool (strict)" method="Reinit To Default"() -> ()  [unwired: 3 in, 3 out]
  n2 = call "initialize_queue.vi"("state"=w1) -> ("error out"=w2:errorcluster, "queue out"=w3:refnum<queue>)  [unwired: 9 in]
  n3 = flat-sequence {
    tunnel: [w10] -> w5
    tunnel: "action buttons" -> [w9]
    tunnel: w2 -> [w7]
    tunnel: w3 -> [w8]
    tunnel: [w848] -> w6
    tunnel: w5 -> [w849]
    frame #0 {
      w11 = T19 {"Shape - t, Color - f"=FALSE, "qsm"={"Webcam image ref"=refnum, "Analyzed image ref"=refnum, "Stop webcam"=FALSE}, " image ref"=refnum, "number img"=0, "ROI Descriptor (Image Mask 1)"={"Global Rectangle"=[109, 72, 345, 284], "Contours"=[{"ID"=enum."External", "Type"=3, "Coordinates"=[109, 72, 345, 284]}]}, "Pattern class"=0, "Color class"=[], "ROI Descriptor COLOR Mask"={"Global Rectangle"=[51, 157, 345, 350], "Contours"=[{"ID"=enum."External", "Type"=5, "Coordinates"=[137, 230, 93, 226, 75, 199, 49, 200, 56, 145, 98, 111, 200, 119, 250, 126, 235, 166, 240, 212, 188, 243, 303, 244, 336, 247, 336, 271, 335, 292, 335, 318, 314, 323, 293, 334, 279, 345, 272, 349, 187, 349, 186, 335, 120, 334, 112, 314, 100, 297, 59, 291, 51, 288, 51, 287]}]}}  # data
      n4 = while {
        shift-right: [w51] -> w10
        shift-left: w7 -> [w56]
        shift-right: [w18] -> _
        shift-left: w11 -> [w32]
        shift-right: [w31] -> _
        shift-left: w9 -> [w30]
        tunnel: w8 -> [w29]
        stop <- w27 stop-if-true
        w34 = 400.0 ("Frequency [Hz]")
        # "define and \ninitialize the \ndata highway\nvalues"
        # "MANIPULATORS"
        # "create the state queue and\nenqueue the initialization task;\nrelease the \"stop\" button"
        # "set front-panel\npolling interval\nin milliseconds"
        # "poll front-panel\nbuttons on each\nloop iteration"
        # "Machine Vision App"
        n5 = xnode "M_PWM"("Duty Cycle"="M_PWM", "Frequency [Hz]"=w34) -> ("error out"=w50:errorcluster)  [unwired: 1 in]
        n6 = xnode "L_PWM"("Duty Cycle"="L_PWM", "Frequency [Hz]"=w34) -> ("error out"=w49:errorcluster)  [unwired: 1 in]
        n7 = xnode "R_PWM"("Duty Cycle"="R_PWM", "Frequency [Hz]"=w34) -> ("error out"=w48:errorcluster)  [unwired: 1 in]
        n8 = Bundle By Name(cluster=w32, "Shape - t, Color - f"=FALSE) -> (w26:T19)
        n9 = Merge Errors(w50, w49, w48) -> (w45:errorcluster)
        n10 = call "dequeue_state.vi"("stop"="Stop", "error in (no error)"=w56, "queue in"=w29) -> ("error out"=w57:errorcluster, "state"=w52:T7, "queue out"=w33:refnum<queue>)  [unwired: 6 in]
        n11 = Wait Until Next ms Multiple(millisecond multiple=u32 25) -> ()  [unwired: 1 out]
        n12 = xnode "Digital output (1 sample)"("Left+ (A/DIO5 (Pin 21))"="Left+", "Right+ (A/DIO7 (Pin 25))"="Right+", "Left- (A/DIO6 (Pin 23))"="Left-", "Right- (A/DIO13 (Pin 26))"="Right-", "error in (no error)"=w45) -> ("error out"=w47:errorcluster)
        n13 = xnode "Digital output (1 sample) 2"("M+ (B/DIO5 (Pin 21))"="M+", "M- (B/DIO6 (Pin 23))"="M-", "G+ (B/DIO7 (Pin 25))"="G+", "G- (B/DIO13 (Pin 26))"="G-", "error in (no error)"=w45) -> ("error out"=w46:errorcluster)
        n14 = case shown="\"(ball) Calculate ROI\"" w52 {
          tunnel: w57 -> [w289 w307 w309 w312 w323 w325 w329 w374 w454 w472 w485 w505 w507 w517 w582 w618 w637 w720 w730 w786 w822 w842]
          tunnel: w33 -> [w290 _ _ _ w322 _ _ _ _ _ _ _ _ _ w581 w616 _ _ _ _ _ _]
          tunnel: [w291 w306 w309 w312 w318 w325 w328 w372 w457 w473 w485 w500 w507 w517 w582 w617 w636 w721 w730 w785 w822 w842] -> w12
          tunnel: w30 -> [w288 w299 w308 w311 w317 w324 w327 w370 w450 w477 w482 w496 w506 w516 w579 w620 w638 w725 w727 w781 w820 w843]
          tunnel: w26 -> [w292 w301 w310 w314 w321 w326 w331 w376 w455 w481 w486 w502 w508 w519 w583 w622 w639 w719 w728 w784 w821 w844]
          tunnel: [w292 w300 w310 w313 w321 w326 w331 w375 w459 w480 w486 w501 w508 w518 w583 w621 w639 w718 w729 w783 w821 w844] -> w19
          tunnel: "mode buttons" -> [_ _ _ _ _ _ _ _ _ _ w484 _ _ _ _ _ _ _ _ _ _ _]
          tunnel: [w288 w299 w308 w311 w317 w324 w327 w370 w450 w477 w482 w496 w506 w516 w579 w619 w638 w725 w727 w781 w820 w843] -> w31
          tunnel: [_ _ _ _ TRUE _ _ _ _ _ _ _ _ _ _ _ _ _ _ _ _ _] -> w27
          frame "(qsm) schedule" {
            # "action buttons"
            # "Schedule tasks -- Use a selector tree (illustrated below), case structures, or other logic to specify state sequences (\"tasks\") to be performed in response to front-panel action buttons and flags set or cleared in other states."
            n15 = Unbundle By Name(w288) -> ("Shape - t, Color - f"=w287:T20)
            n16 = case shown="\"Other\"" w287 {
              tunnel: [w293 w294 w295 w296 w297 w298] -> w286
              frame "Align", Default {
                w293 = T21 [enum."(image) get", enum."(ball) Shape detection", enum."X align", enum."Wait", enum."(image) show", enum."(myRIO) update ports"] items=["(qsm) schedule", "(qsm) initialize", "(qsm) release", "(qsm) clean up", "(qsm) shutdown", "(myRIO) initialize", "(myRIO) clean up", "(myRIO) update ports", "(image) get", "(image) analyze", "(image) show", "(ball) Shape detection", "(ball) Calc ball indx", "(ball) Calculate ROI", "X align", "Wait", "Grab", "(pattern) Find Square", "(pattern) Calculate ROI", "(pattern) Analyze pattern", "(joystick) Joystick control", "Wait for button"]  # default task
              }
              frame "Pattern" {
                w294 = T21 [enum."(image) get", enum."(pattern) Find Square", enum."(pattern) Calculate ROI", enum."(pattern) Analyze pattern", enum."(image) show", enum."(myRIO) update ports", enum."(qsm) schedule"] items=["(qsm) schedule", "(qsm) initialize", "(qsm) release", "(qsm) clean up", "(qsm) shutdown", "(myRIO) initialize", "(myRIO) clean up", "(myRIO) update ports", "(image) get", "(image) analyze", "(image) show", "(ball) Shape detection", "(ball) Calc ball indx", "(ball) Calculate ROI", "X align", "Wait", "Grab", "(pattern) Find Square", "(pattern) Calculate ROI", "(pattern) Analyze pattern", "(joystick) Joystick control", "Wait for button"] ("task")
              }
              frame "Ball" {
                w295 = T21 [enum."(image) get", enum."(ball) Shape detection", enum."(ball) Calculate ROI", enum."(ball) Calc ball indx", enum."(image) analyze", enum."(image) show", enum."(myRIO) update ports", enum."Wait for button"] items=["(qsm) schedule", "(qsm) initialize", "(qsm) release", "(qsm) clean up", "(qsm) shutdown", "(myRIO) initialize", "(myRIO) clean up", "(myRIO) update ports", "(image) get", "(image) analyze", "(image) show", "(ball) Shape detection", "(ball) Calc ball indx", "(ball) Calculate ROI", "X align", "Wait", "Grab", "(pattern) Find Square", "(pattern) Calculate ROI", "(pattern) Analyze pattern", "(joystick) Joystick control", "Wait for button"] ("task")
              }
              frame "Other" {
                w296 = T21 [enum."(image) get", enum."(pattern) Find Square", enum."(pattern) Calculate ROI", enum."(pattern) Analyze pattern", enum."(image) show", enum."Wait for button", enum."(myRIO) update ports", enum."(image) get", enum."(ball) Shape detection", enum."(ball) Calculate ROI", enum."(image) analyze", enum."(image) show", enum."Wait for button", enum."(myRIO) update ports"] items=["(qsm) schedule", "(qsm) initialize", "(qsm) release", "(qsm) clean up", "(qsm) shutdown", "(myRIO) initialize", "(myRIO) clean up", "(myRIO) update ports", "(image) get", "(image) analyze", "(image) show", "(ball) Shape detection", "(ball) Calc ball indx", "(ball) Calculate ROI", "X align", "Wait", "Grab", "(pattern) Find Square", "(pattern) Calculate ROI", "(pattern) Analyze pattern", "(joystick) Joystick control", "Wait for button"] ("task")
              }
              frame "Clear" {
                w297 = T21 [enum."(qsm) release"] items=["(qsm) schedule", "(qsm) initialize", "(qsm) release", "(qsm) clean up", "(qsm) shutdown", "(myRIO) initialize", "(myRIO) clean up", "(myRIO) update ports", "(image) get", "(image) analyze", "(image) show", "(ball) Shape detection", "(ball) Calc ball indx", "(ball) Calculate ROI", "X align", "Wait", "Grab", "(pattern) Find Square", "(pattern) Calculate ROI", "(pattern) Analyze pattern", "(joystick) Joystick control", "Wait for button"]
              }
              frame "Joystick control" {
                w298 = T21 [enum."(joystick) Joystick control"] items=["(qsm) schedule", "(qsm) initialize", "(qsm) release", "(qsm) clean up", "(qsm) shutdown", "(myRIO) initialize", "(myRIO) clean up", "(myRIO) update ports", "(image) get", "(image) analyze", "(image) show", "(ball) Shape detection", "(ball) Calc ball indx", "(ball) Calculate ROI", "X align", "Wait", "Grab", "(pattern) Find Square", "(pattern) Calculate ROI", "(pattern) Analyze pattern", "(joystick) Joystick control", "Wait for button"]
              }
            }
            n17 = call "enqueue_states.vi"("task"=w286, "error in"=w289, "queue in"=w290) -> ("error out"=w291:errorcluster)  [unwired: 6 in, 1 out]
          }
          frame "(qsm) initialize" {
            w304 = T22 0 items=["Grayscale (U8)", "Grayscale (I16)", "Grayscale (SGL)", "Complex (CSG)", "RGB (U32)", "HSL (U32)", "RGB (U64)", "Grayscale (U16)"] ("Image Type")
            # "Initialize -- Allocate memory for additional image buffers, if necessary, and perform other one-time initialization steps."
            n18 = call "IMAQ Create"("Border Size"=3, "Image Name"="img0", "Image Type"=w304, "error in (no error)"=w307) -> ("New Image"=w302:T5, "error out"=w306:errorcluster)  [unwired: 1 in]
            n19 = Bundle By Name(cluster=w301, "image ref"=w302) -> (w300:T19)
          }
          frame "(qsm) release" {
            # "Release all front-panel action buttons."
          }
          frame "(qsm) clean up" {
            # "Set the \"Stop webcam\" flag"
            # "Clean up -- Set the \"Stop webcam flag\" and perform other necessary clean-up actions."
            n20 = Bundle By Name(cluster=w314, "qsm.Stop webcam"=TRUE) -> (w313:T19)
          }
          frame "(qsm) shutdown" {
            # "deallocate image buffer memory"
            # "stop the loop"
            # "Shutdown -- Release the state queue, free all image buffer memory, and stop the while-loop structure."
            n21 = Release Queue(queue=w322, error in (no error)=w323) -> (error out=w319:errorcluster)  [unwired: 1 in, 2 out]
            n22 = call "Imaq Dispose"("All Images? (No)"=TRUE, "error in (no error)"=w319) -> ("error out"=w318:errorcluster)  [unwired: 4 in]
          }
          frame "(myRIO) initialize" {
            # "Initialize (myRIO) -- Open channels, configure devices, send setup strings to peripherals, etc."
          }
          frame "(myRIO) clean up" {
            w330 = FALSE ("LED3")
            # "clear the onboard LEDs"
            # "Clean up (myRIO) -- Return myRIO devices and external peripherals to inactive states."
            n23 = xnode "LED 3"("LED0"=w330, "LED1"=w330, "LED2"=w330, "LED3"=w330, "error in (no error)"=w329) -> ("error out"=w328:errorcluster)
          }
          frame "(myRIO) update ports" {
            # "show the button state\non the onboard LEDs"
            # "set the flag"
            # "press the onboard button\nto set the \"save image\" flag"
            # "Update ports (myRIO) -- Read and write onboard devices and external peripherals."
            n24 = xnode "Button"("error in (no error)"=w374) -> ("Value"=w371:bool, "error out"=w373:errorcluster)
            n25 = Bundle By Name "Bundle By Name"(cluster=w376, "Shape - t, Color - f"=w371) -> (w375:T19)
            n26 = xnode "LED"("LED0"=w371, "LED1"=w371, "LED2"=w371, "LED3"=w371, "error in (no error)"=w373) -> ("error out"=w372:errorcluster)
          }
          frame "(image) get" {
            # "NOTE:\n1. Use NI-MAX to configure your webcam with the\n     *same* resolution (\"mode\") and attributes as those used \n     to develop your Vision Assistant script, especially if the\n     script depends on absolute ROIs, calibration images, template\n     images, background levels, etc.\n \n     Click \"Save\" to create or update the camera configuration files\n     on the target.\n\n2. Open the Vision Acquisition Express VI above and then\n     select \"Reset to Defaults\" to read the camera configuration\n     files created/updated by NI-MAX in the previous step."
            # "webcam image buffer is\ncreated during the first\ncall of the Vision\nAcquisition Express VI"
            # "Get image -- Retrieve a single webcam image frame and optionally flip the image right side up."
            n27 = Unbundle By Name(w455) -> ("qsm.Stop webcam"=w453:bool)
            n28 = call "Vision Acquisition"("Stop (F)"=w453, "error in"=w454) -> ("Image Out"=w452:T5, "error out"=w451:errorcluster)  [unwired: 22 in, 2 out]
            n29 = case shown="False" FALSE {
              tunnel: w452 -> [w461 w465]
              tunnel: [w461 w464] -> w458
              tunnel: w451 -> [w460 w463]
              tunnel: [w460 w462] -> w457
              frame False {
                # "use webcam image as-is"
              }
              frame True {
                w466 = u32 2 items=["Horizontal", "Vertical", "Central", "1st Diagonal", "2nd Diagonal"] ("Type of Symmetry")
                # "flip image when using\ntable-top camera stand"
                n30 = call "IMAQ Symmetry"("error in (no error)"=w463, "Type of Symmetry"=w466, "Image Src"=w465) -> ("error out"=w462:errorcluster, "Image Dst Out"=w464:T5)  [unwired: 2 in]
              }
            }
            n31 = Bundle By Name(cluster=w455, "qsm.Webcam image ref"=w458) -> (w459:T19)
          }
          frame "(image) analyze" {
            # "Color analyze"
            # "analyzed image buffer is\ncreated during the first\ncall of the Vision\nAssistant Express VI *only*\nwhen \"Create Destination\nImage\" option is enabled"
            # "Analyze image -- Analyze the webcam image with a Vision Assistant script."
            n32 = Unbundle By Name "Unbundle By Name"(w481) -> ("Color class"=w471:i32[], "qsm.Webcam image ref"=w476:T5)
            n33 = call "Vision Assistant2"("Image In"=w476, "ROI Descriptor (Color Classification 1)"="ROI Descriptor COLOR Mask", "ROI Descriptor (Image Mask 1)"="ROI Descriptor COLOR Mask", "error in"=w472) -> ("Image Out"=w475:T5, "Classes (Color Classification 1)"=w474:string[], "error out"=w473:errorcluster)  [unwired: 21 in]
            n34 = local read "Ball index"() -> (w469:i32)
            n35 = Index Array(array=w474, index=0) -> (element=w478:string)
            n36 = Decimal String To Number(string=w478) -> (number=w470:i32)  [unwired: 2 in, 1 out]
            "Color" <- w470
            n37 = Replace Array Subset(array=w471, new element=w470, index=w469) -> (w468:i32[])
            n38 = Bundle By Name "Bundle By Name"(cluster=w481, "qsm.Analyzed image ref"=w475, "Color class"=w468) -> (w480:T19)
          }
          frame "(image) show" {
            # "Show image -- Select from among the available image buffers to show on the main image display; use a selector tree or case structure."
            n39 = Unbundle By Name "Unbundle By Name"(w484) -> ("show analyzed"=w483:bool)
            n40 = Unbundle By Name "Unbundle By Name"(w486) -> ("qsm.Analyzed image ref"=w489:T5, "qsm.Webcam image ref"=w488:T5)
            n41 = Select(t=w489, s=w483, f=w488) -> (s? t:f=→"image display":T5)
          }
          frame "(ball) Shape detection" {
            # "Shape detection"
            # "Expansion State A"
            n42 = Unbundle By Name(w502) -> ("qsm.Webcam image ref"=w504:T5)
            n43 = call "Vision Assistant"("Image In"=w504, "error in"=w505, "Circle Descriptor (Shape Detection 1)"="Circle Descriptor (Shape Detection 1)") -> ("Image Out"=w503:T5, "error out"=w500:errorcluster, "Circles Calibrated (Shape Detection 1)"=w498:T2, "Number of Matches (Shape Detection 1)"=→"Number of Matches (Shape Detection 1)":i32)  [unwired: 21 in]
            "Circles Calibrated (Shape Detection 1)" <- w498
            n44 = Index Array(array=w498, index=0) -> (element=w494:T23)
            n45 = Unbundle By Name(w494) -> ("Position"=w493:cluster{"X":sgl, "Y":sgl}, "Radius"=→"CircleRadius":dbl)
            n46 = Unbundle(w493) -> ("X"=→"curX":sgl, "Y"=→"curY":sgl)
            n47 = Bundle By Name(cluster=w502, "qsm.Analyzed image ref"=w503) -> (w501:T19)
          }
          frame "(ball) Calc ball indx" {
            n48 = local read "Number of Matches (Shape Detection 1)"() -> (w510:i32)
            n49 = Greater Than 0?(x=w510) -> (x > 0?=w509:bool)
            n50 = case shown="True" w509 {
              frame False {
              }
              frame True {
                n51 = local read "Number of Matches (Shape Detection 1)"() -> (w512:i32)
                n52 = Less?(x="Ball index", y=w512) -> (x < y?=w511:bool)
                n53 = case shown="True" w511 {
                  frame False {
                  }
                  frame True {
                    n54 = local read "Ball index"() -> (w515:i32)
                    n55 = Increment(x=w515) -> (x+1=w514:i32)
                    n56 = local write "Ball index"(w514) -> ()
                  }
                }
              }
            }
          }
          frame "(ball) Calculate ROI" {
            n57 = local read "Number of Matches (Shape Detection 1)"() -> (w520:i32)
            n58 = Greater Than 0?(x=w520) -> (x > 0?=w521:bool)
            n59 = case shown="True" w521 {
              tunnel: [w528 w547] -> w518
              tunnel: w519 -> [w528 w547]
              frame False {
                w534 = 0 ("index")
                w539 = 0 ("index")
                # "\"Black screen\", if no balls found"
                n60 = local read "ROI Descriptor COLOR Mask"() -> (w523:T1)
                n61 = local read "Ball index"() -> (w529:i32)
                n62 = Unbundle By Name(w523) -> ("Global Rectangle"=w524:i32[], "Contours"=w525:T24)
                n63 = Index Array(array=w525, index=w529) -> (element=w532:T25)
                n64 = Unbundle By Name(w532) -> ("Coordinates"=w533:i32[])
                n65 = Replace Array Subset(array=w524, new element #1=w539, index #1=0 ("index"), new element #2=w539, index #2=1 ("index"), new element #3=w539, index #3=2 ("index"), new element #4=w539, index #4=3 ("index")) -> (w527:i32[])
                n66 = Replace Array Subset(array=w533, new element #1=w534, index #1=0 ("index"), new element #2=w534, index #2=1 ("index"), new element #3=w534, index #3=2 ("index"), new element #4=w534, index #4=3 ("index")) -> (w530:i32[])
                n67 = Bundle By Name(cluster=w532, "Coordinates"=w530) -> (w531:T25)
                n68 = Replace Array Subset(array=w525, new element=w531, index=w529) -> (w526:T24)
                n69 = Bundle By Name(cluster=w523, "Global Rectangle"=w527, "Contours"=w526) -> (w522:T1)
                n70 = local write "ROI Descriptor COLOR Mask"(w522) -> ()
              }
              frame True {
                w544 = 0 ("index")
                n71 = local read "Circles Calibrated (Shape Detection 1)"() -> (w578:T2)
                n72 = local read "ROI Descriptor COLOR Mask"() -> (w546:T1)
                n73 = Index Array(array=w578, index=w544) -> (element=w577:T23)
                n74 = Unbundle By Name(w577) -> ("Position"=w576:cluster{"X":sgl, "Y":sgl}, "Radius"=w545:dbl)
                "Radius (circle)" <- w545
                n75 = Divide(x=w545, y="divider (circle)") -> (x/y=w565:dbl)
                n76 = Unbundle(w576) -> ("X"=w575:sgl, "Y"=w574:sgl)
                n77 = Unbundle By Name(w546) -> ("Global Rectangle"=w563:i32[], "Contours"=w552:T24)
                n78 = Index Array(array=w552, index=w544) -> (element=w550:T25)
                n79 = Unbundle By Name(w550) -> ("Coordinates"=w557:i32[])
                n80 = Subtract(x=w575, y=w565) -> (x-y=w573:dbl)
                n81 = Subtract(x=w574, y=w565) -> (x-y=w572:dbl)
                n82 = Add(x=w575, y=w565) -> (x+y=w570:dbl)
                n83 = Add(x=w574, y=w565) -> (x+y=w571:dbl)
                n84 = To Long Integer(number=w573) -> (32bit integer=w556:i32)
                "x0 (circle)" <- w556
                n85 = To Long Integer(number=w572) -> (32bit integer=w555:i32)
                "y0 (circle)" <- w555
                n86 = To Long Integer(number=w570) -> (32bit integer=w554:i32)
                "x1 (circle)" <- w554
                n87 = To Long Integer(number=w571) -> (32bit integer=w553:i32)
                "y1 (circle)" <- w553
                n88 = local write "ROI Descriptor COLOR Mask"(w546) -> ()
                n89 = Replace Array Subset(array=w563, new element #1=w556, index #1=0 ("index"), new element #2=w555, index #2=1 ("index"), new element #3=w554, index #3=2 ("index"), new element #4=w553, index #4=3 ("index")) -> (w562:i32[])
                n90 = Replace Array Subset(array=w557, new element #1=w556, index #1=0 ("index"), new element #2=w555, index #2=1 ("index"), new element #3=w554, index #3=2 ("index"), new element #4=w553, index #4=3 ("index")) -> (w548:i32[])
                n91 = Bundle By Name(cluster=w550, "Coordinates"=w548) -> (w549:T25)
                n92 = Replace Array Subset(array=w552, new element=w549, index=w544) -> (w551:T24)
                n93 = Bundle By Name(cluster=w546, "Global Rectangle"=w562, "Contours"=w551) -> ()  [unwired: 1 out]
              }
            }
          }
          frame "X align" {
            # "Align"
            # "Expansion State B"
            n94 = case shown="True" "Align X - t, Y - f" {
              tunnel: w581 -> [w585 w601]
              frame False {
                # "Bck"
                # "Fwd"
                # "Y align"
                n95 = local read "curY"() -> (w593:sgl)
                n96 = local read "Range"() -> (w588:dbl)
                n97 = Subtract(x="defY", y=w593) -> (x-y=w587:dbl)
                n98 = Multiply(x=w588, y=-1.0) -> (x*y=w586:dbl)
                n99 = Greater?(x=w587, y=w588) -> (0:w589:bool)
                n100 = Less?(x=w587, y=w586) -> (x < y?=w590:bool)
                n101 = Not Or(1:w590, 2:w589) -> (0:w591:bool)
                "Y is in range" <- w591
                n102 = case shown="True" w591 {
                  tunnel: w585 -> [_ w594]
                  frame False {
                  }
                  frame True {
                    n103 = local read "X is in range"() -> (w595:bool)
                    n104 = case shown="True" w595 {
                      tunnel: w594 -> [_ w597]
                      frame False {
                        n105 = local write "Align X - t, Y - f"(TRUE ("X - t, Y - f")) -> ()
                      }
                      frame True {
                        w598 = T21 [enum."Wait", enum."(image) get", enum."(myRIO) clean up", enum."(qsm) shutdown"] items=["(qsm) schedule", "(qsm) initialize", "(qsm) release", "(qsm) clean up", "(qsm) shutdown", "(myRIO) initialize", "(myRIO) clean up", "(myRIO) update ports", "(image) get", "(image) analyze", "(image) show", "(ball) Shape detection", "(ball) Calc ball indx", "(ball) Calculate ROI", "X align", "Wait", "Grab", "(pattern) Find Square", "(pattern) Calculate ROI", "(pattern) Analyze pattern", "(joystick) Joystick control", "Wait for button"] ("task")
                        n106 = call "enqueue_states.vi"("task"=w598, "queue in"=w597) -> ()  [unwired: 7 in, 2 out]
                      }
                    }
                  }
                }
                n107 = local write "Left-"(w590) -> ()
                n108 = local write "Left+"(w589) -> ()
                n109 = local write "Right+"(w589) -> ()
                n110 = local write "Right-"(w590) -> ()
              }
              frame True {
                # "X align"
                # "Right"
                # "Left"
                n111 = local read "curX"() -> (w602:sgl)
                n112 = Subtract(x="defX", y=w602) -> (x-y=w609:dbl)
                n113 = Multiply(x="Range", y=-1.0) -> (x*y=w608:dbl)
                n114 = Greater?(x=w609, y="Range") -> (0:w599:bool)
                n115 = Less?(x=w609, y=w608) -> (x < y?=w600:bool)
                n116 = Not(x=w600) -> (.not. x?=w605:bool)
                n117 = Not(x=w600) -> (.not. x?=w606:bool)
                n118 = And(x=w606, y=w605) -> (x .and. y?=w604:bool)
                "X is in range" <- w604
                n119 = case shown="True" w604 {
                  tunnel: w601 -> [_ w611]
                  frame False {
                  }
                  frame True {
                    n120 = local read "Y is in range"() -> (w612:bool)
                    n121 = case shown="True" w612 {
                      tunnel: w611 -> [_ w614]
                      frame False {
                        n122 = local write "Align X - t, Y - f"(FALSE ("X - t, Y - f")) -> ()
                      }
                      frame True {
                        w615 = T21 [enum."Wait", enum."(image) get", enum."(myRIO) clean up", enum."(qsm) shutdown"] items=["(qsm) schedule", "(qsm) initialize", "(qsm) release", "(qsm) clean up", "(qsm) shutdown", "(myRIO) initialize", "(myRIO) clean up", "(myRIO) update ports", "(image) get", "(image) analyze", "(image) show", "(ball) Shape detection", "(ball) Calc ball indx", "(ball) Calculate ROI", "X align", "Wait", "Grab", "(pattern) Find Square", "(pattern) Calculate ROI", "(pattern) Analyze pattern", "(joystick) Joystick control", "Wait for button"] ("task")
                        n123 = call "enqueue_states.vi"("task"=w615, "queue in"=w614) -> ()  [unwired: 7 in, 2 out]
                      }
                    }
                  }
                }
                n124 = local write "Left-"(w599) -> ()
                n125 = local write "Left+"(w600) -> ()
                n126 = local write "Right+"(w599) -> ()
                n127 = local write "Right-"(w600) -> ()
              }
            }
          }
          frame "Wait" {
            w626 = FALSE
            # "Expansion State D"
            n128 = local read "X is in range"() -> (w624:bool)
            n129 = local read "Y is in range"() -> (w623:bool)
            n130 = local write "Left-"(w626) -> ()
            n131 = local write "Left+"(w626) -> ()
            n132 = local write "Right+"(w626) -> ()
            n133 = local write "Right-"(w626) -> ()
            n134 = And(x=w624, y=w623) -> (x .and. y?=w625:bool)
            n135 = case shown="True" w625 {
              tunnel: w622 -> [w629 w634]
              tunnel: [w629 w634] -> w621
              tunnel: w620 -> [w628 w635]
              tunnel: [w628 w635] -> w619
              tunnel: w618 -> [w627 w630]
              tunnel: [w627 w633] -> w617
              tunnel: w616 -> [_ w631]
              frame False {
              }
              frame True {
                w632 = T21 [enum."(image) get", enum."(image) analyze", enum."(image) show", enum."(myRIO) update ports", enum."Grab", enum."Wait"] items=["(qsm) schedule", "(qsm) initialize", "(qsm) release", "(qsm) clean up", "(qsm) shutdown", "(myRIO) initialize", "(myRIO) clean up", "(myRIO) update ports", "(image) get", "(image) analyze", "(image) show", "(ball) Shape detection", "(ball) Calc ball indx", "(ball) Calculate ROI", "X align", "Wait", "Grab", "(pattern) Find Square", "(pattern) Calculate ROI", "(pattern) Analyze pattern", "(joystick) Joystick control", "Wait for button"] ("task")
                n136 = call "enqueue_states.vi"("task"=w632, "error in"=w630, "queue in"=w631) -> ("error out"=w633:errorcluster)  [unwired: 6 in, 1 out]
              }
            }
          }
          frame "Grab" {
            # "Expansion State E"
            n137 = flat-sequence {
              tunnel: w637 -> [w642]
              tunnel: [w641] -> w636
              frame #0 {
                n138 = xnode "M_PWM 2"("Duty Cycle"=0.5, "Frequency [Hz]"=400.0, "error in (no error)"=w642) -> ("error out"=w643:errorcluster)
                n139 = xnode "Digital output (1 sample) 3"("M+ (B/DIO5 (Pin 21))"="M+ (onGrab)", "error in (no error)"=w643) -> ("error out"=w641:errorcluster)
                n140 = Wait (ms)(milliseconds to wait="grab time (ms)") -> ()  [unwired: 1 out]
              }
            }
          }
          frame "(pattern) Find Square" {
            # "analyzed image buffer is\ncreated during the first\ncall of the Vision\nAssistant Express VI *only*\nwhen \"Create Destination\nImage\" option is enabled"
            # "Expansion State F"
            n141 = Unbundle By Name "Unbundle By Name"(w719) -> ("qsm.Webcam image ref"=w724:T5)
            n142 = call "Vision Assistant3"("Image In"=w724, "error in"=w720) -> ("Image Out"=w717:T5, "error out"=w721:errorcluster, "Calibrated Matches (Geometric Matching 1)"=→"Calibrated Matches (Geometric Matching 1)":T3[], "Number of Matches (Geometric Matching 1)"=→"Number of Matches (Geometric Matching 1)":i32)  [unwired: 22 in]
            n143 = Bundle By Name(cluster=w719, "qsm.Analyzed image ref"=w717) -> (w718:T19)
          }
          frame "(pattern) Calculate ROI" {
            # "Expansion State G"
            n144 = local read "Number of Matches (Geometric Matching 1)"() -> (w726:i32)
            n145 = Greater Than 0?(x=w726) -> (x > 0?=w731:bool)
            n146 = case shown="True" w731 {
              tunnel: [w733 w774] -> w729
              tunnel: w728 -> [w732 w773]
              frame False {
                w734 = 0 ("index")
                # "\"Black screen\", if no squares found"
                n147 = Unbundle By Name(w732) -> ("ROI Descriptor (Image Mask 1).Contours"=w741:T24)
                n148 = Index Array(array=w741, index=0) -> (element=w744:T25)
                n149 = Unbundle By Name(w744) -> ("Coordinates"=w743:i32[])
                n150 = Replace Array Subset(array=w743, new element #1=w734, index #1=0 ("index"), new element #2=w734, index #2=1 ("index"), new element #3=w734, index #3=2 ("index"), new element #4=w734, index #4=3 ("index")) -> (w745:i32[])
                n151 = Bundle By Name(cluster=w744, "Coordinates"=w745) -> (w746:T25)
                n152 = Replace Array Subset(array=w741, new element=w746, index=0) -> (w742:T24)
                n153 = Bundle By Name(cluster=w732, "ROI Descriptor (Image Mask 1).Contours"=w742) -> (w733:T19)
              }
              frame True {
                n154 = local read "Scale"() -> (w749:sgl)
                n155 = local read "Calibrated Matches (Geometric Matching 1)"() -> (w778:T3[])
                n156 = Index Array(array=w778, index=0) -> (element=w776:T3)
                n157 = Unbundle By Name(w776) -> ("Position"=w775:cluster{"x":sgl, "y":sgl}, "Scale"=→"Scale":sgl)
                n158 = Divide(x=w749, y="y") -> (x/y=w748:sgl)
                n159 = Unbundle(w775) -> ("x"=w768:sgl, "y"=w767:sgl)
                n160 = Unbundle By Name(w773) -> ("ROI Descriptor (Image Mask 1).Contours"=w771:T24)
                n161 = Index Array(array=w771, index=0) -> (element=w760:T25)
                n162 = Unbundle By Name(w760) -> ("Coordinates"=w762:i32[])
                n163 = Subtract(x=w768, y=w748) -> (x-y=w766:sgl)
                n164 = Subtract(x=w767, y=w748) -> (x-y=w765:sgl)
                n165 = Add(x=w768, y=w748) -> (x+y=w763:sgl)
                n166 = Add(x=w767, y=w748) -> (x+y=w764:sgl)
                n167 = To Long Integer(number=w766) -> (32bit integer=w757:i32)
                "x0" <- w757
                n168 = To Long Integer(number=w765) -> (32bit integer=w756:i32)
                "y0" <- w756
                n169 = To Long Integer(number=w763) -> (32bit integer=w755:i32)
                "x1" <- w755
                n170 = To Long Integer(number=w764) -> (32bit integer=w754:i32)
                "y1" <- w754
                n171 = Replace Array Subset(array=w762, new element #1=w757, index #1=0 ("index"), new element #2=w756, index #2=1 ("index"), new element #3=w755, index #3=2 ("index"), new element #4=w754, index #4=3 ("index")) -> (w759:i32[])
                n172 = Bundle By Name(cluster=w760, "Coordinates"=w759) -> (w758:T25)
                n173 = Replace Array Subset(array=w771, new element=w758, index=0) -> (w770:T24)
                n174 = Bundle By Name(cluster=w773, "ROI Descriptor (Image Mask 1).Contours"=w770) -> (w774:T19)
              }
            }
          }
          frame "(pattern) Analyze pattern" {
            n175 = Unbundle By Name(w784) -> ("qsm.Webcam image ref"=w788:T5, "ROI Descriptor (Image Mask 1)"=w782:T1)
            n176 = call "Vision Assistant4"("Image In"=w788, "error in"=w786, "ROI Descriptor (Image Mask 1)"=w782, "ROI Descriptor (Particle Classification 1)"=w782) -> ("Image Out"=w787:T5, "error out"=w785:errorcluster, "Class (Particle Classification 1)"=w780:string)  [unwired: 21 in]
            "Class (Particle Classification 1)" <- w780
            n177 = Decimal String To Number(string=w780) -> (number=w779:i32)  [unwired: 2 in, 1 out]
            n178 = Bundle By Name(cluster=w784, "qsm.Analyzed image ref"=w787, "Pattern class"=w779) -> (w783:T19)
          }
          frame "(joystick) Joystick control" {
            # "Cross (-1 - none; 0 - up; 90 - right; 180 - down; 270 - left)"
            n179 = shared-variable "My Computer\\KeyLibrary.lvlib\\Cross"() -> (w819:i32)  [unwired: 1 in, 1 out]
            n180 = shared-variable "My Computer\\KeyLibrary.lvlib\\A"() -> (w814:bool)  [unwired: 1 in, 1 out]
            n181 = shared-variable "My Computer\\KeyLibrary.lvlib\\B"() -> (w813:bool)  [unwired: 1 in, 1 out]
            n182 = shared-variable "My Computer\\KeyLibrary.lvlib\\X"() -> (w812:bool)  [unwired: 1 in, 1 out]
            n183 = shared-variable "My Computer\\KeyLibrary.lvlib\\Y"() -> (w811:bool)  [unwired: 1 in, 1 out]
            n184 = Equal?(x=w819, y=0) -> (x = y?=w806:bool)
            n185 = Equal?(x=w819, y=90) -> (x = y?=w805:bool)
            n186 = Equal?(x=w819, y=180) -> (x = y?=w804:bool)
            n187 = Equal?(x=w819, y=270) -> (x = y?=w803:bool)
            n188 = Or(x=w803, y=w812) -> (x .or. y?=w815:bool)
            n189 = local write "G-"(w815) -> ()
            n190 = Or(x=w806, y=w811) -> (x .or. y?=w818:bool)
            n191 = Or(x=w804, y=w814) -> (x .or. y?=w817:bool)
            n192 = local write "M+"(w818) -> ()
            n193 = local write "M-"(w817) -> ()
            n194 = Or(x=w805, y=w813) -> (x .or. y?=w816:bool)
            n195 = local write "G+"(w816) -> ()
            n196 = shared-variable "My Computer\\KeyLibrary.lvlib\\RS X"() -> (w790:i32)  [unwired: 1 in, 1 out]
            n197 = shared-variable "My Computer\\KeyLibrary.lvlib\\LS Y"() -> (w791:i32)  [unwired: 1 in, 1 out]
            n198 = Absolute Value(x=w791) -> (abs(x)=w802:i32)
            n199 = Absolute Value(x=w790) -> (abs(x)=w801:i32)
            n200 = Greater?(x=w802, y=w801) -> (0:w792:bool)
            n201 = case shown="False" w792 {
              tunnel: w791 -> [_ w824]
              tunnel: w790 -> [w823 _]
              tunnel: [w823 w824] -> w789
              frame False {
              }
              frame True {
              }
            }
            n202 = Greater?(x=w789, y=3000) -> (0:w797:bool)
            n203 = Less?(x=w789, y=-3000) -> (x < y?=w795:bool)
            n204 = Select(t=w802, s=w792, f=w801) -> (s? t:f=w794:i32)
            n205 = To Double Precision Float(number=w794) -> (double precision float=w800:dbl)
            n206 = case shown="False" w792 {
              tunnel: w797 -> [w825 w834]
              tunnel: w795 -> [w826 w833]
              frame False {
                # "X"
                n207 = case shown="False" w826 {
                  selector: w826 -> [_ w827]
                  frame False {
                  }
                  frame True {
                    n208 = Not(x=w827) -> (.not. x?=w828:bool)
                    n209 = Not(x=w827) -> (.not. x?=w829:bool)
                    n210 = local write "Right+"(w827) -> ()
                    n211 = local write "Right-"(w829) -> ()
                    n212 = local write "Left+"(w828) -> ()
                    n213 = local write "Left-"(w827) -> ()
                  }
                }
                n214 = case shown="False" w825 {
                  selector: w825 -> [_ w830]
                  frame False {
                  }
                  frame True {
                    n215 = Not(x=w830) -> (.not. x?=w832:bool)
                    n216 = Not(x=w830) -> (.not. x?=w831:bool)
                    n217 = local write "Right+"(w831) -> ()
                    n218 = local write "Right-"(w830) -> ()
                    n219 = local write "Left+"(w830) -> ()
                    n220 = local write "Left-"(w832) -> ()
                  }
                }
              }
              frame True {
                # "Y"
                n221 = case shown="True" w833 {
                  selector: w833 -> [_ w835]
                  frame False {
                  }
                  frame True {
                    n222 = Not(x=w835) -> (.not. x?=w837:bool)
                    n223 = Not(x=w835) -> (.not. x?=w836:bool)
                    n224 = local write "Right+"(w837) -> ()
                    n225 = local write "Right-"(w835) -> ()
                    n226 = local write "Left+"(w836) -> ()
                    n227 = local write "Left-"(w835) -> ()
                  }
                }
                n228 = case shown="True" w834 {
                  selector: w834 -> [_ w838]
                  frame False {
                  }
                  frame True {
                    n229 = Not(x=w838) -> (.not. x?=w839:bool)
                    n230 = Not(x=w838) -> (.not. x?=w840:bool)
                    n231 = local write "Left+"(w838) -> ()
                    n232 = local write "Left-"(w840) -> ()
                    n233 = local write "Right+"(w838) -> ()
                    n234 = local write "Right-"(w839) -> ()
                  }
                }
              }
            }
            n235 = Divide(x=w800, y="sensivity") -> (x/y=w793:dbl)
            n236 = local write "R_PWM"(w793) -> ()
            n237 = local write "L_PWM"(w793) -> ()
          }
          frame "Wait for button" {
            n238 = while {
              stop <- w847 stop-if-true
              n239 = local read "Stop"() -> (w846:bool)
              n240 = Or(x="Look at ball", y=w846) -> (x .or. y?=w847:bool)
            }
            n241 = local write "Look at ball"(FALSE ("Look at ball")) -> ()
          }
        }
        n242 = Merge Errors(w47, w46) -> (w24:errorcluster)
        n243 = xnode "LED"("LED0"="x = y?", "error in (no error)"=w24) -> ("error out"=w23:errorcluster)
        n244 = Unbundle By Name(w19) -> ("Pattern class"=w22:i32, "Color class"=w16:i32[])
        n245 = Merge Errors(w12, w23) -> (w51:errorcluster)
        n246 = Index Array(array=w16, index=0) -> (element=w15:i32)
        n247 = Equal?(x=w22, y=w15) -> (x = y?=w13:bool)
        n248 = local read "Number of Matches (Shape Detection 1)"() -> (w21:i32)
        n249 = local write "x = y?"(w13) -> ()
        n250 = Greater Than 0?(x=w21) -> (x > 0?=w20:bool)
        n251 = case shown="True" w20 {
          tunnel: [w61 w69] -> w18
          tunnel: w19 -> [w60 w69]
          frame False {
            n252 = local read "Ball index"() -> (w59:i32)
            n253 = Increment(x=w59) -> (x+1=w58:i32)
            n254 = for {
              N: w58 -> [w63]
              shift-right: [w68] -> w61
              shift-left: w60 -> [w67]
              w64 = -1 ("Color")
              n255 = Unbundle By Name(w67) -> ("Color class"=w66:i32[])
              n256 = Decrement(x=w63) -> (x-1=w62:i32)
              n257 = local write "Color"(w64) -> ()
              n258 = Replace Array Subset(array=w66, new element=w64, index=w62) -> (w65:i32[])
              n259 = Bundle By Name(cluster=w67, "Color class"=w65) -> (w68:T19)
            }
          }
          frame True {
          }
        }
      }
    }
    frame #1 {
      w850 = FALSE ("X is in range")
      n260 = local write "Align X - t, Y - f"(TRUE ("Align X - t, Y - f")) -> ()
      n261 = call <vilib>:"Simple Error Handler.vi"("error in (no error)"=w849) -> ("error out"=w848:errorcluster)  [unwired: 4 in, 4 out]
      "error out" <- w848
      n262 = local write "X is in range"(w850) -> ()
      n263 = local write "Y is in range"(w850) -> ()
      n264 = local write "Stop"(w850) -> ()
      n265 = local write "Look at ball"(w850) -> ()
      n266 = local write "x = y?"(w850) -> ()
    }
  }
  n267 = call <vilib>:"Reset myRIO.vi"("error in (no error)"=w6) -> ()  [unwired: 10 in, 1 out]
